vi "Treat Command.vi"(8 "error in (no error)":errorcluster, 11 "Channel in":refnum<class "Channel.lvclass">) -> (0 "error out":errorcluster, 3 "Channel out":refnum<class "Channel.lvclass">)   [LabVIEW 2018, in "Channel.lvclass"]
uses:
  Channel.lvclass
  Channel.lvclass/Channel.ctl
  CCDCamera/CCDCamera.lvclass/CCDCamera.ctl
  Cooler/Cooler.lvclass/Cooler.ctl
  Save Image/Save Image.lvclass/Save Image.ctl
  CCDCamera/CCDCamera.lvclass
  Cooler/Cooler.lvclass
  State Machine/State Machine.lvclass
  RxTx/RxTx.lvclass
  Image Constructor/Image Constructor.lvclass
  Interface/Interface.lvclass
  Save Image/Save Image.lvclass
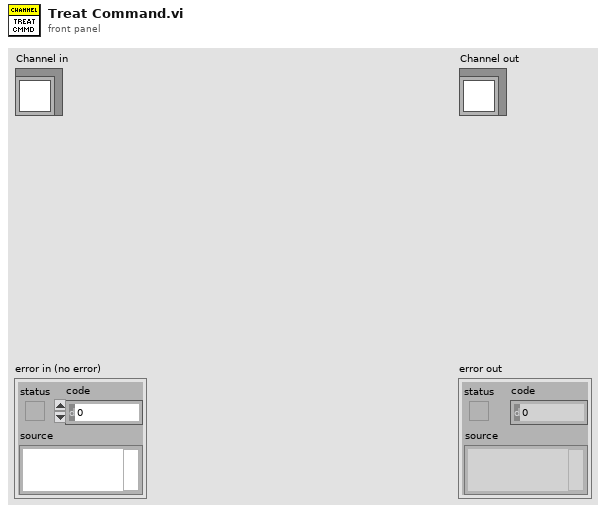
[diagram p1: front panel]
types:
  T1 = cluster{"Initialization":bool, "Serial Number":u16}
  T2 = cluster{"Current Temperature":i16, "Temperatue Status":string}
  T3 = cluster{"Exposure Time":sgl, "Pre-amp gain":u8, "Readout Rate":u8, "EM Mode":u8, "EM Gain":u16, "Binning":u16, "Initial Line":u16, "Initial Cloumn":u16, "Final Line":u16, "Final Column":u16, "Kinetic Series Length":u32, "Shutter Mode":u8, "Cooler ON/OFF":u16, "Temperature":i8, "Image Name":string, "Image Path":string, "# Images":u32}
  T4 = cluster{"Image Path":string, "Image Name":string, "Exposure Time":sgl, "Pre-amp gain":u8, "Readout Rate":u8, "EM Mode":u8, "EM Gain":u16, "Binning":u16, "Initial Line":u16, "Initial Cloumn":u16, "Final Line":u16, "Final Column":u16, "Kinetic Series Length":u32, "Shutter Mode":u8, "Cooler ON/OFF":u16, "Temperature":i8}
  T5 = cluster{"Initial Line":u16, "Initial Column":u16, "Final Line ":u16, "Final Column":u16, "Binning":u16, "Kinetic Series Length":u16, "Image Name":string, "Image Path":string}
  T6 = cluster{"Exposure Time":sgl, "EM Gain":u16, "Binning":u16, "Initial Line":u16, "Initial Cloumn":u16, "Final Line":u16, "Final Column":u16, "Kinetic Series Length":u32, "Shutter Mode":u8, "Pre-amp gain":u8, "Readout Rate":u8, "EM Mode":u8}
  T7 = cluster{"Exposure Time":sgl, "Pre-amp gain":u8, "Readout Rate":u8, "EM Mode":u8, "EM Gain":u16, "Binning":u16, "Initial Line":u16, "Initial Cloumn":u16, "Final Line":u16, "Final Column":u16, "Kinetic Series Length":u32, "Shutter Mode":u8, "Cooler ON/OFF":u16, "Temperature":i8, "Image Name":string, "Image Path":string, "#Images":u32}
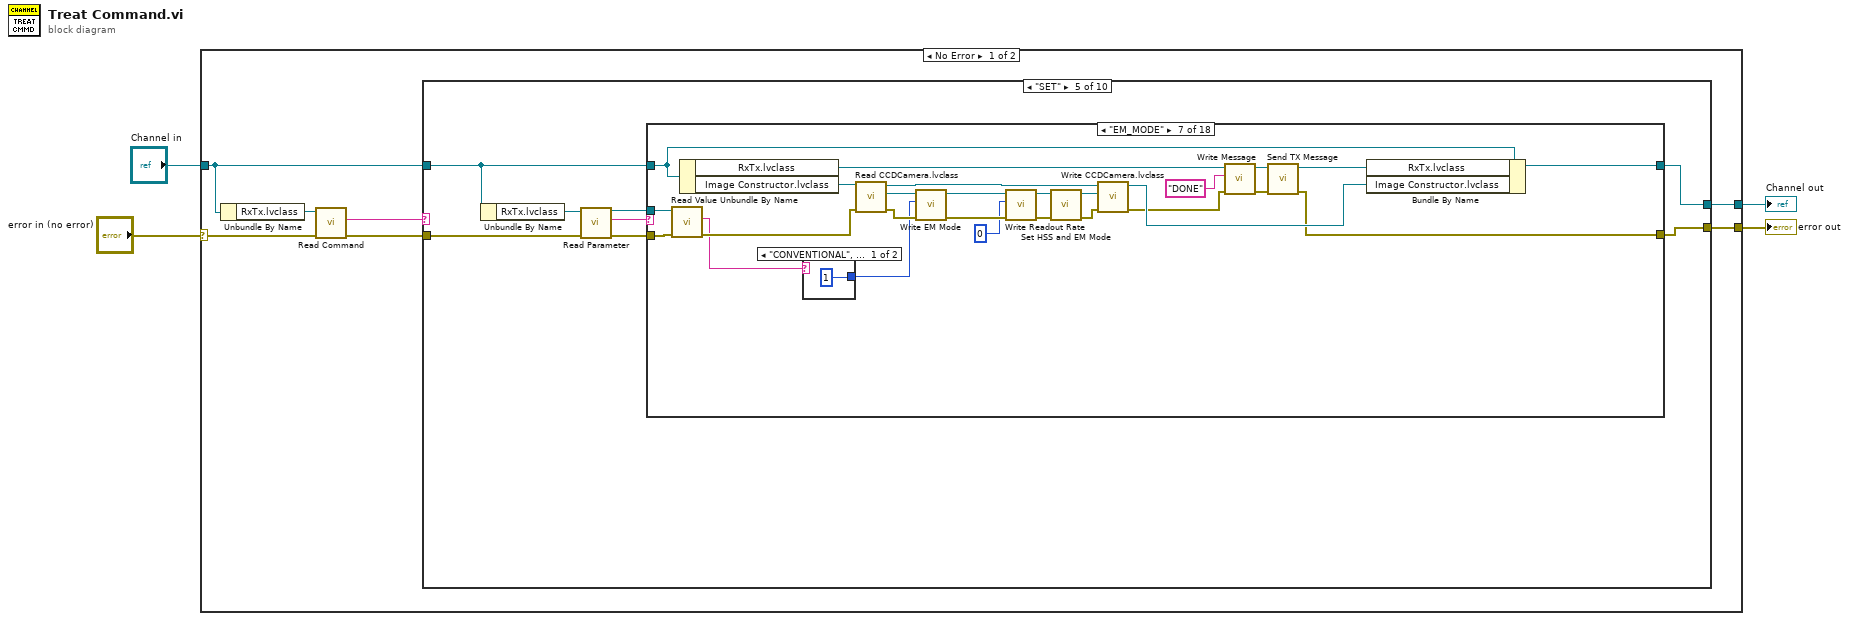
[diagram p0: block diagram]
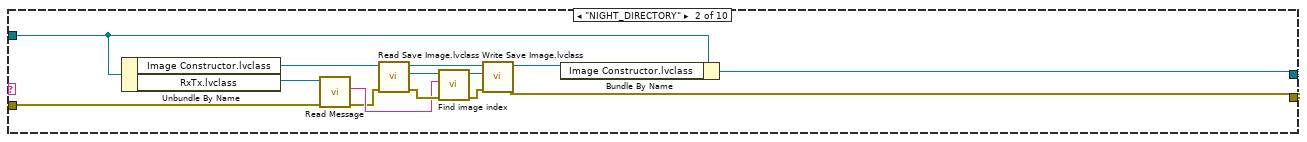
[diagram p3: hidden frame]
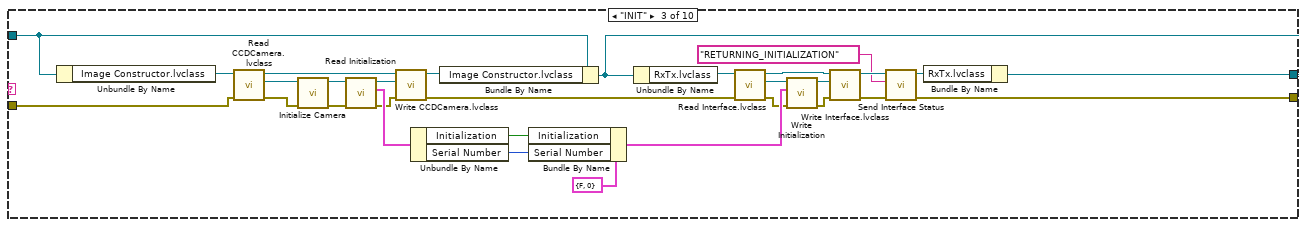
[diagram p4: hidden frame]
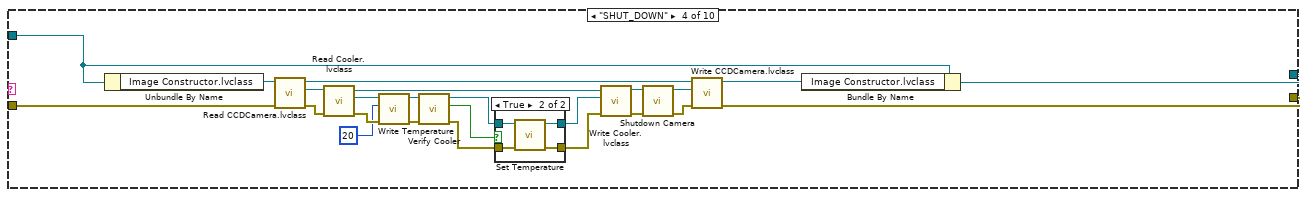
[diagram p5: hidden frame]
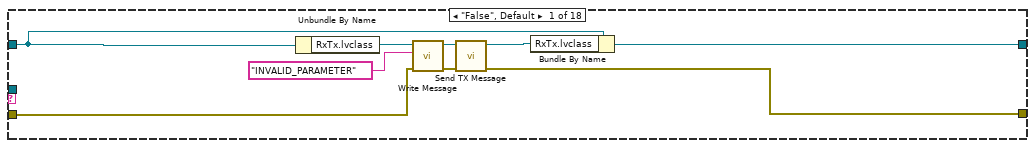
[diagram p7: hidden frame]
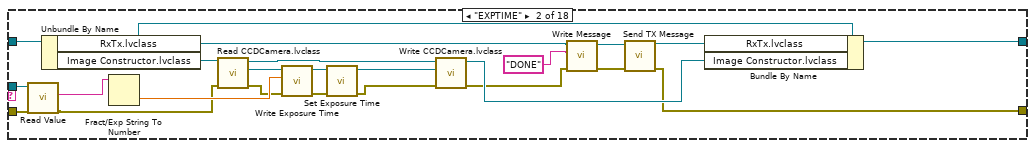
[diagram p8: hidden frame]
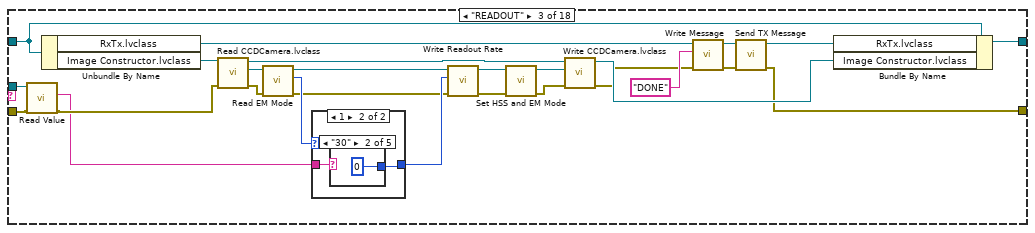
[diagram p9: hidden frame]
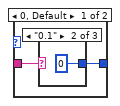
[diagram p10: hidden frame]
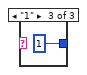
[diagram p12: hidden frame]
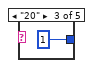
[diagram p14: hidden frame]
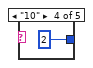
[diagram p15: hidden frame]
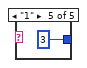
[diagram p16: hidden frame]
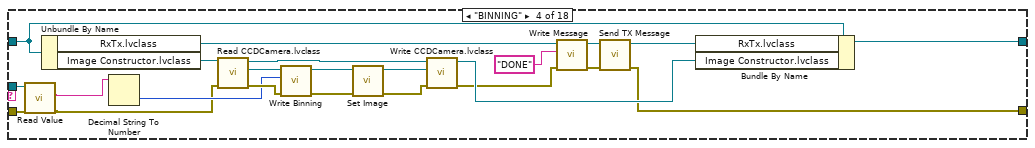
[diagram p17: hidden frame]
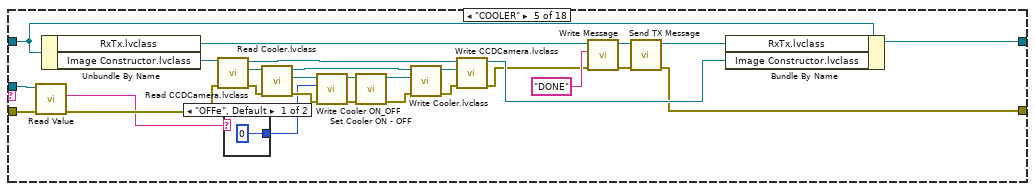
[diagram p18: hidden frame]
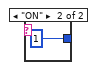
[diagram p19: hidden frame]
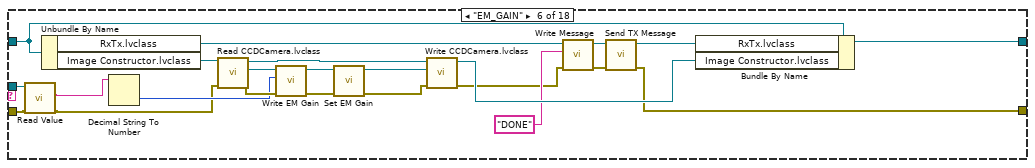
[diagram p20: hidden frame]
diagram:
  n1 = case shown="No Error" "error in (no error)" {
    selector: "error in (no error)" -> [w10 w888]
    tunnel: [w5 w888] -> w3
    tunnel: [w7 w887] -> w1
    tunnel: "Channel in" -> [w8 w887]
    frame No Error {
      n2 = Unbundle By Name(w8) -> ("RxTx.lvclass"=w11:refnum<class "RxTx.lvclass">)
      n3 = call "Read Command.vi"("error in (no error)"=w10, "RxTx in"=w11) -> ("error out"=w6:errorcluster, "Command"=w9:string)  [unwired: 7 in, 1 out]
      n4 = case shown="\"SET\"" w9 {
        tunnel: w8 -> [w13 w16 w31 w60 w90 w518 w769 w802 w841 w885]
        tunnel: [w13 w14 w29 w59 w89 w516 w766 w801 w839 w883] -> w7
        tunnel: w6 -> [w12 w17 w30 w61 w91 w517 w767 w803 w840 w881]
        tunnel: [w12 w15 w28 w58 w88 w515 w765 w800 w838 w882] -> w5
        frame "False", Default {
        }
        frame "NIGHT_DIRECTORY" {
          n5 = Unbundle By Name(w16) -> ("Image Constructor.lvclass"=w26:refnum<class "Image Constructor.lvclass">, "RxTx.lvclass"=w22:refnum<class "RxTx.lvclass">)
          n6 = call "Read Message.vi"("error in (no error)"=w17, "RxTx in"=w22) -> ("error out"=w20:errorcluster, "Message"=w21:string)  [unwired: 7 in, 1 out]
          n7 = call "Read Save Image.lvclass.vi"("error in (no error)"=w20, "Image Constructor in"=w26) -> ("error out"=w24:errorcluster, "Save Image.lvclass"=w23:refnum<class "Save Image.lvclass">, "Image Constructor out"=w27:refnum<class "Image Constructor.lvclass">)  [unwired: 7 in]
          n8 = call "Find image index.vi"("error in (no error)"=w24, "Message"=w21, "Save Image in"=w23) -> ("error out"=w25:errorcluster, "Save Image in"=w19:refnum<class "Save Image.lvclass">)  [unwired: 7 in]
          n9 = call "Write Save Image.lvclass.vi"("error in (no error)"=w25, "Save Image.lvclass"=w19, "Image Constructor in"=w27) -> ("error out"=w15:errorcluster, "Image Constructor out"=w18:refnum<class "Image Constructor.lvclass">)  [unwired: 7 in]
          n10 = Bundle By Name(cluster=w16, "Image Constructor.lvclass"=w18) -> (w14:refnum<class "Channel.lvclass">)
        }
        frame "INIT" {
          n11 = Unbundle By Name(w31) -> ("Image Constructor.lvclass"=w45:refnum<class "Image Constructor.lvclass">)
          n12 = call "Read CCDCamera.lvclass.vi"("error in (no error)"=w30, "Image Constructor in"=w45) -> ("error out"=w47:errorcluster, "CCDCamera.lvclass"=w46:refnum<class "CCDCamera.lvclass">, "Image Constructor out"=w57:refnum<class "Image Constructor.lvclass">)  [unwired: 7 in]
          n13 = call "Initialize Camera.vi"("error in (no error)"=w47, "CCDCamera in"=w46) -> ("error out"=w43:errorcluster, "CCDCamera out"=w44:refnum<class "CCDCamera.lvclass">)  [unwired: 8 in]
          n14 = call "Read Initialization.vi"("error in (no error)"=w43, "CCDCamera in"=w44) -> ("error out"=w52:errorcluster, "Initialization"=w54:T1, "CCDCamera out"=w53:refnum<class "CCDCamera.lvclass">)  [unwired: 7 in]
          n15 = call "Write CCDCamera.lvclass.vi"("error in (no error)"=w52, "CCDCamera.lvclass"=w53, "Image Constructor in"=w57) -> ("error out"=w42:errorcluster, "Image Constructor out"=w56:refnum<class "Image Constructor.lvclass">)  [unwired: 7 in]
          n16 = Unbundle By Name(w54) -> ("Initialization"=w49:bool, "Serial Number"=w48:u16)
          n17 = Bundle By Name(cluster=w31, "Image Constructor.lvclass"=w56) -> (w55:refnum<class "Channel.lvclass">)
          n18 = Bundle By Name(cluster=T1 {"Initialization"=FALSE, "Serial Number"=0} ("Initialization"), "Initialization"=w49, "Serial Number"=w48) -> (w51:T1)
          n19 = Unbundle By Name(w55) -> ("RxTx.lvclass"=w38:refnum<class "RxTx.lvclass">)
          n20 = call "Read Interface.lvclass.vi"("error in (no error)"=w42, "RxTx in"=w38) -> ("error out"=w36:errorcluster, "Interface.lvclass"=w40:refnum<class "Interface.lvclass">, "RxTx out"=w37:refnum<class "RxTx.lvclass">)  [unwired: 7 in]
          n21 = call "Write Initialization.vi"("error in (no error)"=w36, "Initialization"=w51, "Interface in"=w40) -> ("error out"=w41:errorcluster, "Interface out"=w39:refnum<class "Interface.lvclass">)  [unwired: 7 in]
          n22 = call "Write Interface.lvclass.vi"("error in (no error)"=w41, "Interface.lvclass"=w39, "RxTx in"=w37) -> ("error out"=w33:errorcluster, "RxTx out"=w34:refnum<class "RxTx.lvclass">)  [unwired: 7 in]
          n23 = call "Send Interface Status.vi"("error in (no error)"=w33, "Message"="RETURNING_INITIALIZATION", "RxTx in"=w34) -> ("error out"=w28:errorcluster, "RxTx out"=w35:refnum<class "RxTx.lvclass">)  [unwired: 7 in]
          n24 = Bundle By Name(cluster=w55, "RxTx.lvclass"=w35) -> (w29:refnum<class "Channel.lvclass">)
        }
        frame "SHUT_DOWN" {
          n25 = Unbundle By Name(w60) -> ("Image Constructor.lvclass"=w63:refnum<class "Image Constructor.lvclass">)
          n26 = call "Read CCDCamera.lvclass.vi"("error in (no error)"=w61, "Image Constructor in"=w63) -> ("error out"=w65:errorcluster, "CCDCamera.lvclass"=w64:refnum<class "CCDCamera.lvclass">, "Image Constructor out"=w80:refnum<class "Image Constructor.lvclass">)  [unwired: 7 in]
          n27 = call-dynamic "Read Cooler.lvclass.vi"("error in (no error)"=w65, "CCDCamera in"=w64) -> ("error out"=w68:errorcluster, "Cooler.lvclass"=w67:refnum<class "Cooler.lvclass">, "CCDCamera out"=w66:refnum<class "CCDCamera.lvclass">)  [unwired: 7 in]
          n28 = call-dynamic "Write Temperature.vi"("error in (no error)"=w68, "Temperature"=20, "Cooler in"=w67) -> ("error out"=w70:errorcluster, "Cooler out"=w69:refnum<class "Cooler.lvclass">)  [unwired: 7 in]
          n29 = call "Verify Cooler.vi"("error in (no error)"=w70, "Cooler in"=w69) -> ("error out"=w73:errorcluster, "coolerStatus"=w71:bool, "Cooler out"=w72:refnum<class "Cooler.lvclass">)  [unwired: 7 in]
          n30 = case shown="True" w71 {
            tunnel: w72 -> [w83 w87]
            tunnel: w73 -> [w82 w86]
            tunnel: [w82 w85] -> w75
            tunnel: [w83 w84] -> w74
            frame False {
            }
            frame True {
              n31 = call "Set Temperature.vi"("error in (no error)"=w86, "Cooler in"=w87) -> ("error out"=w85:errorcluster, "Cooler out"=w84:refnum<class "Cooler.lvclass">)  [unwired: 8 in]
            }
          }
          n32 = call-dynamic "Write Cooler.lvclass.vi"("error in (no error)"=w75, "Cooler.lvclass"=w74, "CCDCamera in"=w66) -> ("error out"=w76:errorcluster, "CCDCamera out"=w77:refnum<class "CCDCamera.lvclass">)  [unwired: 7 in]
          n33 = call "Shutdown Camera.vi"("error in (no error)"=w76, "CCDCamera in"=w77) -> ("error out"=w79:errorcluster, "CCDCamera out"=w78:refnum<class "CCDCamera.lvclass">)  [unwired: 8 in]
          n34 = call "Write CCDCamera.lvclass.vi"("error in (no error)"=w79, "CCDCamera.lvclass"=w78, "Image Constructor in"=w80) -> ("error out"=w58:errorcluster, "Image Constructor out"=w81:refnum<class "Image Constructor.lvclass">)  [unwired: 7 in]
          n35 = Bundle By Name(cluster=w60, "Image Constructor.lvclass"=w81) -> (w59:refnum<class "Channel.lvclass">)
        }
        frame "SET" {
          n36 = Unbundle By Name(w90) -> ("RxTx.lvclass"=w92:refnum<class "RxTx.lvclass">)
          n37 = call "Read Parameter.vi"("error in (no error)"=w91, "RxTx in"=w92) -> ("error out"=w94:errorcluster, "Parameter"=w93:string, "RxTx out"=w95:refnum<class "RxTx.lvclass">)  [unwired: 7 in]
          n38 = case shown="\"EM_MODE\"" w93 {
            tunnel: [w103 w127 w153 w186 w214 w239 w265 w290 w313 w336 w359 w379 w399 w427 w451 w477 w500 w504] -> w89
            tunnel: w90 -> [w104 w126 w152 w185 w213 w238 w264 w289 w312 w335 w358 w378 w398 w426 w450 w476 w499 w512]
            tunnel: [w98 w109 w142 w169 w202 w225 w252 w274 w297 w322 w344 w367 w389 w417 w438 w463 w486 w501] -> w88
            tunnel: w94 -> [w97 w119 w148 w178 w209 w231 w258 w282 w305 w328 w351 w374 w393 w422 w444 w468 w492 w513]
            tunnel: w95 -> [_ w117 w147 w177 w207 w230 w257 w281 w304 w327 w350 w373 w394 w421 w443 w469 w491 w514]
            frame "False", Default {
              n39 = Unbundle By Name(w104) -> ("RxTx.lvclass"=w100:refnum<class "RxTx.lvclass">)
              n40 = call "Write Message.vi"("error in (no error)"=w97, "Message"="INVALID_PARAMETER", "RxTx in"=w100) -> ("error out"=w102:errorcluster, "RxTx out"=w101:refnum<class "RxTx.lvclass">)  [unwired: 7 in]
              n41 = call "Send TX Message.vi"("error in (no error)"=w102, "RxTx in"=w101) -> ("error out"=w98:errorcluster, "RxTx out"=w99:refnum<class "RxTx.lvclass">)  [unwired: 8 in]
              n42 = Bundle By Name(cluster=w104, "RxTx.lvclass"=w99) -> (w103:refnum<class "Channel.lvclass">)
            }
            frame "EXPTIME" {
              n43 = call "Read Value.vi"("error in (no error)"=w119, "RxTx in"=w117) -> ("error out"=w118:errorcluster, "Value"=w116:string)  [unwired: 7 in, 1 out]
              n44 = Unbundle By Name(w126) -> ("RxTx.lvclass"=w115:refnum<class "RxTx.lvclass">, "Image Constructor.lvclass"=w125:refnum<class "Image Constructor.lvclass">)
              n45 = Fract/Exp String To Number(string=w116) -> (number=w123:dbl)  [unwired: 3 in, 1 out]
              n46 = call "Read CCDCamera.lvclass.vi"("error in (no error)"=w118, "Image Constructor in"=w125) -> ("error out"=w122:errorcluster, "CCDCamera.lvclass"=w124:refnum<class "CCDCamera.lvclass">, "Image Constructor out"=w121:refnum<class "Image Constructor.lvclass">)  [unwired: 7 in]
              n47 = call "Write Exposure Time.vi"("error in (no error)"=w122, "Exposure Time"=w123, "CCDCamera in"=w124) -> ("error out"=w106:errorcluster, "CCDCamera out"=w108:refnum<class "CCDCamera.lvclass">)  [unwired: 7 in]
              n48 = call "Set Exposure Time.vi"("error in (no error)"=w106, "CCDCamera in"=w108) -> ("error out"=w105:errorcluster, "CCDCamera out"=w107:refnum<class "CCDCamera.lvclass">)  [unwired: 8 in]
              n49 = call "Write CCDCamera.lvclass.vi"("error in (no error)"=w105, "CCDCamera.lvclass"=w107, "Image Constructor in"=w121) -> ("error out"=w114:errorcluster, "Image Constructor out"=w120:refnum<class "Image Constructor.lvclass">)  [unwired: 7 in]
              n50 = call "Write Message.vi"("error in (no error)"=w114, "Message"="DONE", "RxTx in"=w115) -> ("error out"=w112:errorcluster, "RxTx out"=w111:refnum<class "RxTx.lvclass">)  [unwired: 7 in]
              n51 = call "Send TX Message.vi"("error in (no error)"=w112, "RxTx in"=w111) -> ("error out"=w109:errorcluster, "RxTx out"=w110:refnum<class "RxTx.lvclass">)  [unwired: 8 in]
              n52 = Bundle By Name(cluster=w126, "RxTx.lvclass"=w110, "Image Constructor.lvclass"=w120) -> (w127:refnum<class "Channel.lvclass">)
            }
            frame "READOUT" {
              n53 = call "Read Value.vi"("error in (no error)"=w148, "RxTx in"=w147) -> ("error out"=w146:errorcluster, "Value"=w131:string)  [unwired: 7 in, 1 out]
              n54 = Unbundle By Name(w152) -> ("RxTx.lvclass"=w140:refnum<class "RxTx.lvclass">, "Image Constructor.lvclass"=w151:refnum<class "Image Constructor.lvclass">)
              n55 = call "Read CCDCamera.lvclass.vi"("error in (no error)"=w146, "Image Constructor in"=w151) -> ("error out"=w133:errorcluster, "CCDCamera.lvclass"=w134:refnum<class "CCDCamera.lvclass">, "Image Constructor out"=w150:refnum<class "Image Constructor.lvclass">)  [unwired: 7 in]
              n56 = call "Read EM Mode.vi"("error in (no error)"=w133, "CCDCamera in"=w134) -> ("error out"=w129:errorcluster, "EM Mode"=w132:u8, "CCDCamera out"=w128:refnum<class "CCDCamera.lvclass">)  [unwired: 7 in]
              n57 = case shown="1" w132 {
                tunnel: w131 -> [w155 w159]
                tunnel: [w154 w158] -> w130
                frame 0, Default {
                  n58 = case shown="\"0.1\"" w155 {
                    tunnel: [_ 0 1] -> w154
                    frame "False", Default {
                    }
                    frame "0.1" {
                    }
                    frame "1" {
                    }
                  }
                }
                frame 1 {
                  n59 = case shown="\"30\"" w159 {
                    tunnel: [_ 0 1 2 3] -> w158
                    frame "False", Default {
                    }
                    frame "30" {
                    }
                    frame "20" {
                    }
                    frame "10" {
                    }
                    frame "1" {
                    }
                  }
                }
              }
              n60 = call "Write Readout Rate.vi"("error in (no error)"=w129, "Readout Rate"=w130, "CCDCamera in"=w128) -> ("error out"=w137:errorcluster, "CCDCamera out"=w138:refnum<class "CCDCamera.lvclass">)  [unwired: 7 in]
              n61 = call "Set HSS and EM Mode.vi"("error in (no error)"=w137, "CCDCamera in"=w138) -> ("error out"=w136:errorcluster, "CCDCamera out"=w135:refnum<class "CCDCamera.lvclass">)  [unwired: 8 in]
              n62 = call "Write CCDCamera.lvclass.vi"("error in (no error)"=w136, "CCDCamera.lvclass"=w135, "Image Constructor in"=w150) -> ("error out"=w139:errorcluster, "Image Constructor out"=w149:refnum<class "Image Constructor.lvclass">)  [unwired: 7 in]
              n63 = call "Write Message.vi"("error in (no error)"=w139, "Message"="DONE", "RxTx in"=w140) -> ("error out"=w141:errorcluster, "RxTx out"=w145:refnum<class "RxTx.lvclass">)  [unwired: 7 in]
              n64 = call "Send TX Message.vi"("error in (no error)"=w141, "RxTx in"=w145) -> ("error out"=w142:errorcluster, "RxTx out"=w143:refnum<class "RxTx.lvclass">)  [unwired: 8 in]
              n65 = Bundle By Name(cluster=w152, "RxTx.lvclass"=w143, "Image Constructor.lvclass"=w149) -> (w153:refnum<class "Channel.lvclass">)
            }
            frame "BINNING" {
              n66 = call "Read Value.vi"("error in (no error)"=w178, "RxTx in"=w177) -> ("error out"=w176:errorcluster, "Value"=w175:string)  [unwired: 7 in, 1 out]
              n67 = Unbundle By Name(w185) -> ("RxTx.lvclass"=w171:refnum<class "RxTx.lvclass">, "Image Constructor.lvclass"=w184:refnum<class "Image Constructor.lvclass">)
              n68 = Decimal String To Number(string=w175) -> (number=w179:i32)  [unwired: 2 in, 1 out]
              n69 = call "Read CCDCamera.lvclass.vi"("error in (no error)"=w176, "Image Constructor in"=w184) -> ("error out"=w180:errorcluster, "CCDCamera.lvclass"=w181:refnum<class "CCDCamera.lvclass">, "Image Constructor out"=w183:refnum<class "Image Constructor.lvclass">)  [unwired: 7 in]
              n70 = call "Write Binning.vi"("error in (no error)"=w180, "Binning"=w179, "CCDCamera in"=w181) -> ("error out"=w164:errorcluster, "CCDCamera out"=w167:refnum<class "CCDCamera.lvclass">)  [unwired: 7 in]
              n71 = call "Set Image.vi"("error in (no error)"=w164, "CCDCamera in"=w167) -> ("error out"=w165:errorcluster, "CCDCamera out"=w166:refnum<class "CCDCamera.lvclass">)  [unwired: 8 in]
              n72 = call "Write CCDCamera.lvclass.vi"("error in (no error)"=w165, "CCDCamera.lvclass"=w166, "Image Constructor in"=w183) -> ("error out"=w168:errorcluster, "Image Constructor out"=w182:refnum<class "Image Constructor.lvclass">)  [unwired: 7 in]
              n73 = call "Write Message.vi"("error in (no error)"=w168, "Message"="DONE", "RxTx in"=w171) -> ("error out"=w174:errorcluster, "RxTx out"=w173:refnum<class "RxTx.lvclass">)  [unwired: 7 in]
              n74 = call "Send TX Message.vi"("error in (no error)"=w174, "RxTx in"=w173) -> ("error out"=w169:errorcluster, "RxTx out"=w170:refnum<class "RxTx.lvclass">)  [unwired: 8 in]
              n75 = Bundle By Name(cluster=w185, "RxTx.lvclass"=w170, "Image Constructor.lvclass"=w182) -> (w186:refnum<class "Channel.lvclass">)
            }
            frame "COOLER" {
              n76 = call "Read Value.vi"("error in (no error)"=w209, "RxTx in"=w207) -> ("error out"=w208:errorcluster, "Value"=w188:string)  [unwired: 7 in, 1 out]
              n77 = Unbundle By Name(w213) -> ("RxTx.lvclass"=w204:refnum<class "RxTx.lvclass">, "Image Constructor.lvclass"=w212:refnum<class "Image Constructor.lvclass">)
              n78 = call "Read CCDCamera.lvclass.vi"("error in (no error)"=w208, "Image Constructor in"=w212) -> ("error out"=w198:errorcluster, "CCDCamera.lvclass"=w199:refnum<class "CCDCamera.lvclass">, "Image Constructor out"=w211:refnum<class "Image Constructor.lvclass">)  [unwired: 7 in]
              n79 = case shown="\"OFFe\", Default" w188 {
                tunnel: [0 1] -> w187
                frame "OFFe", Default {
                }
                frame "ON" {
                }
              }
              n80 = call-dynamic "Read Cooler.lvclass.vi"("error in (no error)"=w198, "CCDCamera in"=w199) -> ("error out"=w190:errorcluster, "Cooler.lvclass"=w191:refnum<class "Cooler.lvclass">, "CCDCamera out"=w189:refnum<class "CCDCamera.lvclass">)  [unwired: 7 in]
              n81 = call "Write Cooler ON_OFF.vi"("error in (no error)"=w190, "Cooler ON/OFF"=w187, "Cooler in"=w191) -> ("error out"=w192:errorcluster, "Cooler out"=w193:refnum<class "Cooler.lvclass">)  [unwired: 7 in]
              n82 = call "Set Cooler ON - OFF.vi"("error in (no error)"=w192, "Cooler in"=w193) -> ("error out"=w194:errorcluster, "Cooler out"=w195:refnum<class "Cooler.lvclass">)  [unwired: 8 in]
              n83 = call-dynamic "Write Cooler.lvclass.vi"("error in (no error)"=w194, "Cooler.lvclass"=w195, "CCDCamera in"=w189) -> ("error out"=w196:errorcluster, "CCDCamera out"=w197:refnum<class "CCDCamera.lvclass">)  [unwired: 7 in]
              n84 = call "Write CCDCamera.lvclass.vi"("error in (no error)"=w196, "CCDCamera.lvclass"=w197, "Image Constructor in"=w211) -> ("error out"=w200:errorcluster, "Image Constructor out"=w210:refnum<class "Image Constructor.lvclass">)  [unwired: 7 in]
              n85 = call "Write Message.vi"("error in (no error)"=w200, "Message"="DONE", "RxTx in"=w204) -> ("error out"=w206:errorcluster, "RxTx out"=w205:refnum<class "RxTx.lvclass">)  [unwired: 7 in]
              n86 = call "Send TX Message.vi"("error in (no error)"=w206, "RxTx in"=w205) -> ("error out"=w202:errorcluster, "RxTx out"=w203:refnum<class "RxTx.lvclass">)  [unwired: 8 in]
              n87 = Bundle By Name(cluster=w213, "RxTx.lvclass"=w203, "Image Constructor.lvclass"=w210) -> (w214:refnum<class "Channel.lvclass">)
            }
            frame "EM_GAIN" {
              n88 = call "Read Value.vi"("error in (no error)"=w231, "RxTx in"=w230) -> ("error out"=w229:errorcluster, "Value"=w228:string)  [unwired: 7 in, 1 out]
              n89 = Unbundle By Name(w238) -> ("RxTx.lvclass"=w223:refnum<class "RxTx.lvclass">, "Image Constructor.lvclass"=w237:refnum<class "Image Constructor.lvclass">)
              n90 = Decimal String To Number(string=w228) -> (number=w232:i32)  [unwired: 2 in, 1 out]
              n91 = call "Read CCDCamera.lvclass.vi"("error in (no error)"=w229, "Image Constructor in"=w237) -> ("error out"=w233:errorcluster, "CCDCamera.lvclass"=w234:refnum<class "CCDCamera.lvclass">, "Image Constructor out"=w236:refnum<class "Image Constructor.lvclass">)  [unwired: 7 in]
              n92 = call "Write EM Gain.vi"("error in (no error)"=w233, "EM Gain"=w232, "CCDCamera in"=w234) -> ("error out"=w220:errorcluster, "CCDCamera out"=w219:refnum<class "CCDCamera.lvclass">)  [unwired: 7 in]
              n93 = call "Set EM Gain.vi"("error in (no error)"=w220, "CCDCamera in"=w219) -> ("error out"=w217:errorcluster, "CCDCamera out"=w218:refnum<class "CCDCamera.lvclass">)  [unwired: 8 in]
              n94 = call "Write CCDCamera.lvclass.vi"("error in (no error)"=w217, "CCDCamera.lvclass"=w218, "Image Constructor in"=w236) -> ("error out"=w221:errorcluster, "Image Constructor out"=w235:refnum<class "Image Constructor.lvclass">)  [unwired: 7 in]
              n95 = call "Write Message.vi"("error in (no error)"=w221, "Message"="DONE", "RxTx in"=w223) -> ("error out"=w227:errorcluster, "RxTx out"=w226:refnum<class "RxTx.lvclass">)  [unwired: 7 in]
              n96 = call "Send TX Message.vi"("error in (no error)"=w227, "RxTx in"=w226) -> ("error out"=w225:errorcluster, "RxTx out"=w224:refnum<class "RxTx.lvclass">)  [unwired: 8 in]
              n97 = Bundle By Name(cluster=w238, "RxTx.lvclass"=w224, "Image Constructor.lvclass"=w235) -> (w239:refnum<class "Channel.lvclass">)
            }
            frame "EM_MODE" {
              n98 = call "Read Value.vi"("error in (no error)"=w258, "RxTx in"=w257) -> ("error out"=w256:errorcluster, "Value"=w246:string)  [unwired: 7 in, 1 out]
              n99 = Unbundle By Name(w264) -> ("RxTx.lvclass"=w250:refnum<class "RxTx.lvclass">, "Image Constructor.lvclass"=w263:refnum<class "Image Constructor.lvclass">)
              n100 = case shown="\"CONVENTIONAL\", Default" w246 {
                tunnel: [1 0] -> w245
                frame "CONVENTIONAL", Default {
                }
                frame "EM" {
                }
              }
              n101 = call "Read CCDCamera.lvclass.vi"("error in (no error)"=w256, "Image Constructor in"=w263) -> ("error out"=w259:errorcluster, "CCDCamera.lvclass"=w260:refnum<class "CCDCamera.lvclass">, "Image Constructor out"=w262:refnum<class "Image Constructor.lvclass">)  [unwired: 7 in]
              n102 = call "Write EM Mode.vi"("error in (no error)"=w259, "EM Mode"=w245, "CCDCamera in"=w260) -> ("error out"=w241:errorcluster, "CCDCamera out"=w244:refnum<class "CCDCamera.lvclass">)  [unwired: 7 in]
              n103 = call "Write Readout Rate.vi"("error in (no error)"=w241, "Readout Rate"=0, "CCDCamera in"=w244) -> ("error out"=w242:errorcluster, "CCDCamera out"=w243:refnum<class "CCDCamera.lvclass">)  [unwired: 7 in]
              n104 = call "Set HSS and EM Mode.vi"("error in (no error)"=w242, "CCDCamera in"=w243) -> ("error out"=w247:errorcluster, "CCDCamera out"=w248:refnum<class "CCDCamera.lvclass">)  [unwired: 8 in]
              n105 = call "Write CCDCamera.lvclass.vi"("error in (no error)"=w247, "CCDCamera.lvclass"=w248, "Image Constructor in"=w262) -> ("error out"=w251:errorcluster, "Image Constructor out"=w261:refnum<class "Image Constructor.lvclass">)  [unwired: 7 in]
              n106 = call "Write Message.vi"("error in (no error)"=w251, "Message"="DONE", "RxTx in"=w250) -> ("error out"=w255:errorcluster, "RxTx out"=w254:refnum<class "RxTx.lvclass">)  [unwired: 7 in]
              n107 = call "Send TX Message.vi"("error in (no error)"=w255, "RxTx in"=w254) -> ("error out"=w252:errorcluster, "RxTx out"=w253:refnum<class "RxTx.lvclass">)  [unwired: 8 in]
              n108 = Bundle By Name(cluster=w264, "RxTx.lvclass"=w253, "Image Constructor.lvclass"=w261) -> (w265:refnum<class "Channel.lvclass">)
            }
            frame "FINAL_COLUMN" {
              n109 = call "Read Value.vi"("error in (no error)"=w282, "RxTx in"=w281) -> ("error out"=w280:errorcluster, "Value"=w279:string)  [unwired: 7 in, 1 out]
              n110 = Unbundle By Name(w289) -> ("RxTx.lvclass"=w276:refnum<class "RxTx.lvclass">, "Image Constructor.lvclass"=w288:refnum<class "Image Constructor.lvclass">)
              n111 = Decimal String To Number(string=w279) -> (number=w283:i32)  [unwired: 2 in, 1 out]
              n112 = call "Read CCDCamera.lvclass.vi"("error in (no error)"=w280, "Image Constructor in"=w288) -> ("error out"=w284:errorcluster, "CCDCamera.lvclass"=w285:refnum<class "CCDCamera.lvclass">, "Image Constructor out"=w287:refnum<class "Image Constructor.lvclass">)  [unwired: 7 in]
              n113 = call "Write Final Column.vi"("error in (no error)"=w284, "Final Column"=w283, "CCDCamera in"=w285) -> ("error out"=w270:errorcluster, "CCDCamera out"=w271:refnum<class "CCDCamera.lvclass">)  [unwired: 7 in]
              n114 = call "Set Image.vi"("error in (no error)"=w270, "CCDCamera in"=w271) -> ("error out"=w268:errorcluster, "CCDCamera out"=w269:refnum<class "CCDCamera.lvclass">)  [unwired: 8 in]
              n115 = call "Write CCDCamera.lvclass.vi"("error in (no error)"=w268, "CCDCamera.lvclass"=w269, "Image Constructor in"=w287) -> ("error out"=w273:errorcluster, "Image Constructor out"=w286:refnum<class "Image Constructor.lvclass">)  [unwired: 7 in]
              n116 = call "Write Message.vi"("error in (no error)"=w273, "Message"="DONE", "RxTx in"=w276) -> ("error out"=w278:errorcluster, "RxTx out"=w277:refnum<class "RxTx.lvclass">)  [unwired: 7 in]
              n117 = call "Send TX Message.vi"("error in (no error)"=w278, "RxTx in"=w277) -> ("error out"=w274:errorcluster, "RxTx out"=w275:refnum<class "RxTx.lvclass">)  [unwired: 8 in]
              n118 = Bundle By Name(cluster=w289, "RxTx.lvclass"=w275, "Image Constructor.lvclass"=w286) -> (w290:refnum<class "Channel.lvclass">)
            }
            frame "FINAL_LINE" {
              n119 = call "Read Value.vi"("error in (no error)"=w305, "RxTx in"=w304) -> ("error out"=w303:errorcluster, "Value"=w302:string)  [unwired: 7 in, 1 out]
              n120 = Unbundle By Name(w312) -> ("RxTx.lvclass"=w299:refnum<class "RxTx.lvclass">, "Image Constructor.lvclass"=w311:refnum<class "Image Constructor.lvclass">)
              n121 = Decimal String To Number(string=w302) -> (number=w306:i32)  [unwired: 2 in, 1 out]
              n122 = call "Read CCDCamera.lvclass.vi"("error in (no error)"=w303, "Image Constructor in"=w311) -> ("error out"=w307:errorcluster, "CCDCamera.lvclass"=w308:refnum<class "CCDCamera.lvclass">, "Image Constructor out"=w310:refnum<class "Image Constructor.lvclass">)  [unwired: 7 in]
              n123 = call "Write Final Line.vi"("error in (no error)"=w307, "Final Line"=w306, "CCDCamera in"=w308) -> ("error out"=w293:errorcluster, "CCDCamera out"=w294:refnum<class "CCDCamera.lvclass">)  [unwired: 7 in]
              n124 = call "Set Image.vi"("error in (no error)"=w293, "CCDCamera in"=w294) -> ("error out"=w291:errorcluster, "CCDCamera out"=w292:refnum<class "CCDCamera.lvclass">)  [unwired: 8 in]
              n125 = call "Write CCDCamera.lvclass.vi"("error in (no error)"=w291, "CCDCamera.lvclass"=w292, "Image Constructor in"=w310) -> ("error out"=w296:errorcluster, "Image Constructor out"=w309:refnum<class "Image Constructor.lvclass">)  [unwired: 7 in]
              n126 = call "Write Message.vi"("error in (no error)"=w296, "Message"="DONE", "RxTx in"=w299) -> ("error out"=w301:errorcluster, "RxTx out"=w300:refnum<class "RxTx.lvclass">)  [unwired: 7 in]
              n127 = call "Send TX Message.vi"("error in (no error)"=w301, "RxTx in"=w300) -> ("error out"=w297:errorcluster, "RxTx out"=w298:refnum<class "RxTx.lvclass">)  [unwired: 8 in]
              n128 = Bundle By Name(cluster=w312, "RxTx.lvclass"=w298, "Image Constructor.lvclass"=w309) -> (w313:refnum<class "Channel.lvclass">)
            }
            frame "INITIAL_COLUMN" {
              n129 = call "Read Value.vi"("error in (no error)"=w328, "RxTx in"=w327) -> ("error out"=w326:errorcluster, "Value"=w325:string)  [unwired: 7 in, 1 out]
              n130 = Unbundle By Name(w335) -> ("RxTx.lvclass"=w320:refnum<class "RxTx.lvclass">, "Image Constructor.lvclass"=w334:refnum<class "Image Constructor.lvclass">)
              n131 = Decimal String To Number(string=w325) -> (number=w329:i32)  [unwired: 2 in, 1 out]
              n132 = call "Read CCDCamera.lvclass.vi"("error in (no error)"=w326, "Image Constructor in"=w334) -> ("error out"=w330:errorcluster, "CCDCamera.lvclass"=w331:refnum<class "CCDCamera.lvclass">, "Image Constructor out"=w333:refnum<class "Image Constructor.lvclass">)  [unwired: 7 in]
              n133 = call "Write Initial Cloumn.vi"("error in (no error)"=w330, "Initial Cloumn"=w329, "CCDCamera in"=w331) -> ("error out"=w316:errorcluster, "CCDCamera out"=w317:refnum<class "CCDCamera.lvclass">)  [unwired: 7 in]
              n134 = call "Set Image.vi"("error in (no error)"=w316, "CCDCamera in"=w317) -> ("error out"=w314:errorcluster, "CCDCamera out"=w315:refnum<class "CCDCamera.lvclass">)  [unwired: 8 in]
              n135 = call "Write CCDCamera.lvclass.vi"("error in (no error)"=w314, "CCDCamera.lvclass"=w315, "Image Constructor in"=w333) -> ("error out"=w318:errorcluster, "Image Constructor out"=w332:refnum<class "Image Constructor.lvclass">)  [unwired: 7 in]
              n136 = call "Write Message.vi"("error in (no error)"=w318, "Message"="DONE", "RxTx in"=w320) -> ("error out"=w324:errorcluster, "RxTx out"=w323:refnum<class "RxTx.lvclass">)  [unwired: 7 in]
              n137 = call "Send TX Message.vi"("error in (no error)"=w324, "RxTx in"=w323) -> ("error out"=w322:errorcluster, "RxTx out"=w321:refnum<class "RxTx.lvclass">)  [unwired: 8 in]
              n138 = Bundle By Name(cluster=w335, "RxTx.lvclass"=w321, "Image Constructor.lvclass"=w332) -> (w336:refnum<class "Channel.lvclass">)
            }
            frame "INITIAL_LINE" {
              n139 = call "Read Value.vi"("error in (no error)"=w351, "RxTx in"=w350) -> ("error out"=w349:errorcluster, "Value"=w348:string)  [unwired: 7 in, 1 out]
              n140 = Unbundle By Name(w358) -> ("RxTx.lvclass"=w345:refnum<class "RxTx.lvclass">, "Image Constructor.lvclass"=w357:refnum<class "Image Constructor.lvclass">)
              n141 = Decimal String To Number(string=w348) -> (number=w352:i32)  [unwired: 2 in, 1 out]
              n142 = call "Read CCDCamera.lvclass.vi"("error in (no error)"=w349, "Image Constructor in"=w357) -> ("error out"=w353:errorcluster, "CCDCamera.lvclass"=w354:refnum<class "CCDCamera.lvclass">, "Image Constructor out"=w356:refnum<class "Image Constructor.lvclass">)  [unwired: 7 in]
              n143 = call "Write Initial Line.vi"("error in (no error)"=w353, "Initial Line"=w352, "CCDCamera in"=w354) -> ("error out"=w339:errorcluster, "CCDCamera out"=w340:refnum<class "CCDCamera.lvclass">)  [unwired: 7 in]
              n144 = call "Set Image.vi"("error in (no error)"=w339, "CCDCamera in"=w340) -> ("error out"=w338:errorcluster, "CCDCamera out"=w337:refnum<class "CCDCamera.lvclass">)  [unwired: 8 in]
              n145 = call "Write CCDCamera.lvclass.vi"("error in (no error)"=w338, "CCDCamera.lvclass"=w337, "Image Constructor in"=w356) -> ("error out"=w342:errorcluster, "Image Constructor out"=w355:refnum<class "Image Constructor.lvclass">)  [unwired: 7 in]
              n146 = call "Write Message.vi"("error in (no error)"=w342, "Message"="DONE", "RxTx in"=w345) -> ("error out"=w343:errorcluster, "RxTx out"=w347:refnum<class "RxTx.lvclass">)  [unwired: 7 in]
              n147 = call "Send TX Message.vi"("error in (no error)"=w343, "RxTx in"=w347) -> ("error out"=w344:errorcluster, "RxTx out"=w346:refnum<class "RxTx.lvclass">)  [unwired: 8 in]
              n148 = Bundle By Name(cluster=w358, "RxTx.lvclass"=w346, "Image Constructor.lvclass"=w355) -> (w359:refnum<class "Channel.lvclass">)
            }
            frame "IMAGE_PATH" {
              n149 = call "Read Value.vi"("error in (no error)"=w374, "RxTx in"=w373) -> ("error out"=w372:errorcluster, "Value"=w360:string)  [unwired: 7 in, 1 out]
              n150 = Unbundle By Name(w378) -> ("RxTx.lvclass"=w368:refnum<class "RxTx.lvclass">, "Image Constructor.lvclass"=w377:refnum<class "Image Constructor.lvclass">)
              n151 = call "Read Save Image.lvclass.vi"("error in (no error)"=w372, "Image Constructor in"=w377) -> ("error out"=w361:errorcluster, "Save Image.lvclass"=w362:refnum<class "Save Image.lvclass">, "Image Constructor out"=w376:refnum<class "Image Constructor.lvclass">)  [unwired: 7 in]
              n152 = call "Write Image Path.vi"("error in (no error)"=w361, "Image Path"=w360, "Save Image in"=w362) -> ("error out"=w363:errorcluster, "Save Image out"=w364:refnum<class "Save Image.lvclass">)  [unwired: 7 in]
              n153 = call "Write Save Image.lvclass.vi"("error in (no error)"=w363, "Save Image.lvclass"=w364, "Image Constructor in"=w376) -> ("error out"=w366:errorcluster, "Image Constructor out"=w375:refnum<class "Image Constructor.lvclass">)  [unwired: 7 in]
              n154 = call "Write Message.vi"("error in (no error)"=w366, "Message"="DONE", "RxTx in"=w368) -> ("error out"=w371:errorcluster, "RxTx out"=w370:refnum<class "RxTx.lvclass">)  [unwired: 7 in]
              n155 = call "Send TX Message.vi"("error in (no error)"=w371, "RxTx in"=w370) -> ("error out"=w367:errorcluster, "RxTx out"=w369:refnum<class "RxTx.lvclass">)  [unwired: 8 in]
              n156 = Bundle By Name(cluster=w378, "RxTx.lvclass"=w369, "Image Constructor.lvclass"=w375) -> (w379:refnum<class "Channel.lvclass">)
            }
            frame "IMAGE_NAME" {
              n157 = call "Read Value.vi"("error in (no error)"=w393, "RxTx in"=w394) -> ("error out"=w392:errorcluster, "Value"=w380:string)  [unwired: 7 in, 1 out]
              n158 = Unbundle By Name(w398) -> ("RxTx.lvclass"=w387:refnum<class "RxTx.lvclass">, "Image Constructor.lvclass"=w397:refnum<class "Image Constructor.lvclass">)
              n159 = call "Read Save Image.lvclass.vi"("error in (no error)"=w392, "Image Constructor in"=w397) -> ("error out"=w383:errorcluster, "Save Image.lvclass"=w384:refnum<class "Save Image.lvclass">, "Image Constructor out"=w396:refnum<class "Image Constructor.lvclass">)  [unwired: 7 in]
              n160 = call "Write Image Name.vi"("error in (no error)"=w383, "Image Name"=w380, "Save Image in"=w384) -> ("error out"=w381:errorcluster, "Save Image out"=w382:refnum<class "Save Image.lvclass">)  [unwired: 7 in]
              n161 = call "Write Save Image.lvclass.vi"("error in (no error)"=w381, "Save Image.lvclass"=w382, "Image Constructor in"=w396) -> ("error out"=w386:errorcluster, "Image Constructor out"=w395:refnum<class "Image Constructor.lvclass">)  [unwired: 7 in]
              n162 = call "Write Message.vi"("error in (no error)"=w386, "Message"="DONE", "RxTx in"=w387) -> ("error out"=w391:errorcluster, "RxTx out"=w390:refnum<class "RxTx.lvclass">)  [unwired: 7 in]
              n163 = call "Send TX Message.vi"("error in (no error)"=w391, "RxTx in"=w390) -> ("error out"=w389:errorcluster, "RxTx out"=w388:refnum<class "RxTx.lvclass">)  [unwired: 8 in]
              n164 = Bundle By Name(cluster=w398, "RxTx.lvclass"=w388, "Image Constructor.lvclass"=w395) -> (w399:refnum<class "Channel.lvclass">)
            }
            frame "TEMPERATURE" {
              n165 = call "Read Value.vi"("error in (no error)"=w422, "RxTx in"=w421) -> ("error out"=w420:errorcluster, "Value"=w419:string)  [unwired: 7 in, 1 out]
              n166 = Unbundle By Name(w426) -> ("RxTx.lvclass"=w412:refnum<class "RxTx.lvclass">, "Image Constructor.lvclass"=w425:refnum<class "Image Constructor.lvclass">)
              n167 = Decimal String To Number(string=w419) -> (number=w401:i32)  [unwired: 2 in, 1 out]
              n168 = call "Read CCDCamera.lvclass.vi"("error in (no error)"=w420, "Image Constructor in"=w425) -> ("error out"=w408:errorcluster, "CCDCamera.lvclass"=w409:refnum<class "CCDCamera.lvclass">, "Image Constructor out"=w424:refnum<class "Image Constructor.lvclass">)  [unwired: 7 in]
              n169 = call-dynamic "Read Cooler.lvclass.vi"("error in (no error)"=w408, "CCDCamera in"=w409) -> ("error out"=w406:errorcluster, "Cooler.lvclass"=w407:refnum<class "Cooler.lvclass">, "CCDCamera out"=w400:refnum<class "CCDCamera.lvclass">)  [unwired: 7 in]
              n170 = call-dynamic "Write Temperature.vi"("error in (no error)"=w406, "Temperature"=w401, "Cooler in"=w407) -> ("error out"=w402:errorcluster, "Cooler out"=w403:refnum<class "Cooler.lvclass">)  [unwired: 7 in]
              n171 = call "Set Temperature.vi"("error in (no error)"=w402, "Cooler in"=w403) -> ("error out"=w404:errorcluster, "Cooler out"=w405:refnum<class "Cooler.lvclass">)  [unwired: 8 in]
              n172 = call-dynamic "Write Cooler.lvclass.vi"("error in (no error)"=w404, "Cooler.lvclass"=w405, "CCDCamera in"=w400) -> ("error out"=w410:errorcluster, "CCDCamera out"=w411:refnum<class "CCDCamera.lvclass">)  [unwired: 7 in]
              n173 = call "Write CCDCamera.lvclass.vi"("error in (no error)"=w410, "CCDCamera.lvclass"=w411, "Image Constructor in"=w424) -> ("error out"=w414:errorcluster, "Image Constructor out"=w423:refnum<class "Image Constructor.lvclass">)  [unwired: 7 in]
              n174 = call "Write Message.vi"("error in (no error)"=w414, "Message"="DONE", "RxTx in"=w412) -> ("error out"=w416:errorcluster, "RxTx out"=w418:refnum<class "RxTx.lvclass">)  [unwired: 7 in]
              n175 = call "Send TX Message.vi"("error in (no error)"=w416, "RxTx in"=w418) -> ("error out"=w417:errorcluster, "RxTx out"=w415:refnum<class "RxTx.lvclass">)  [unwired: 8 in]
              n176 = Bundle By Name(cluster=w426, "RxTx.lvclass"=w415, "Image Constructor.lvclass"=w423) -> (w427:refnum<class "Channel.lvclass">)
            }
            frame "SHUTTER" {
              n177 = call "Read Value.vi"("error in (no error)"=w444, "RxTx in"=w443) -> ("error out"=w442:errorcluster, "Value"=w428:string)  [unwired: 7 in, 1 out]
              n178 = Unbundle By Name(w450) -> ("RxTx.lvclass"=w437:refnum<class "RxTx.lvclass">, "Image Constructor.lvclass"=w449:refnum<class "Image Constructor.lvclass">)
              n179 = To Upper Case(1:w428) -> (0:w429:string)
              n180 = case shown="\"CLOSED\", Default" w429 {
                tunnel: [2 1 0] -> w430
                frame "CLOSED", Default {
                }
                frame "OPEN" {
                }
                frame "AUTO" {
                }
              }
              n181 = call "Read CCDCamera.lvclass.vi"("error in (no error)"=w442, "Image Constructor in"=w449) -> ("error out"=w445:errorcluster, "CCDCamera.lvclass"=w446:refnum<class "CCDCamera.lvclass">, "Image Constructor out"=w448:refnum<class "Image Constructor.lvclass">)  [unwired: 7 in]
              n182 = call "Write Shutter Mode.vi"("error in (no error)"=w445, "Shutter Mode"=w430, "CCDCamera in"=w446) -> ("error out"=w433:errorcluster, "CCDCamera out"=w434:refnum<class "CCDCamera.lvclass">)  [unwired: 7 in]
              n183 = call "Set Shutter Mode.vi"("error in (no error)"=w433, "CCDCamera in"=w434) -> ("error out"=w431:errorcluster, "CCDCamera out"=w432:refnum<class "CCDCamera.lvclass">)  [unwired: 8 in]
              n184 = call "Write CCDCamera.lvclass.vi"("error in (no error)"=w431, "CCDCamera.lvclass"=w432, "Image Constructor in"=w448) -> ("error out"=w436:errorcluster, "Image Constructor out"=w447:refnum<class "Image Constructor.lvclass">)  [unwired: 7 in]
              n185 = call "Write Message.vi"("error in (no error)"=w436, "Message"="DONE", "RxTx in"=w437) -> ("error out"=w441:errorcluster, "RxTx out"=w440:refnum<class "RxTx.lvclass">)  [unwired: 7 in]
              n186 = call "Send TX Message.vi"("error in (no error)"=w441, "RxTx in"=w440) -> ("error out"=w438:errorcluster, "RxTx out"=w439:refnum<class "RxTx.lvclass">)  [unwired: 8 in]
              n187 = Bundle By Name(cluster=w450, "RxTx.lvclass"=w439, "Image Constructor.lvclass"=w447) -> (w451:refnum<class "Channel.lvclass">)
            }
            frame "PREAMP" {
              n188 = call "Read Value.vi"("error in (no error)"=w468, "RxTx in"=w469) -> ("error out"=w467:errorcluster, "Value"=w466:string)  [unwired: 7 in, 1 out]
              n189 = Unbundle By Name(w476) -> ("RxTx.lvclass"=w461:refnum<class "RxTx.lvclass">, "Image Constructor.lvclass"=w475:refnum<class "Image Constructor.lvclass">)
              n190 = Decimal String To Number(string=w466) -> (number=w470:i32)  [unwired: 2 in, 1 out]
              n191 = call "Read CCDCamera.lvclass.vi"("error in (no error)"=w467, "Image Constructor in"=w475) -> ("error out"=w471:errorcluster, "CCDCamera.lvclass"=w472:refnum<class "CCDCamera.lvclass">, "Image Constructor out"=w474:refnum<class "Image Constructor.lvclass">)  [unwired: 7 in]
              n192 = call "Write Pre-amp gain.vi"("error in (no error)"=w471, "Pre-amp gain"=w470, "CCDCamera in"=w472) -> ("error out"=w457:errorcluster, "CCDCamera out"=w458:refnum<class "CCDCamera.lvclass">)  [unwired: 7 in]
              n193 = call "Set Pre Amplification.vi"("error in (no error)"=w457, "CCDCamera in"=w458) -> ("error out"=w455:errorcluster, "CCDCamera out"=w456:refnum<class "CCDCamera.lvclass">)  [unwired: 8 in]
              n194 = call "Write CCDCamera.lvclass.vi"("error in (no error)"=w455, "CCDCamera.lvclass"=w456, "Image Constructor in"=w474) -> ("error out"=w460:errorcluster, "Image Constructor out"=w473:refnum<class "Image Constructor.lvclass">)  [unwired: 7 in]
              n195 = call "Write Message.vi"("error in (no error)"=w460, "Message"="DONE", "RxTx in"=w461) -> ("error out"=w465:errorcluster, "RxTx out"=w464:refnum<class "RxTx.lvclass">)  [unwired: 7 in]
              n196 = call "Send TX Message.vi"("error in (no error)"=w465, "RxTx in"=w464) -> ("error out"=w463:errorcluster, "RxTx out"=w462:refnum<class "RxTx.lvclass">)  [unwired: 8 in]
              n197 = Bundle By Name(cluster=w476, "RxTx.lvclass"=w462, "Image Constructor.lvclass"=w473) -> (w477:refnum<class "Channel.lvclass">)
            }
            frame "KSERLEN" {
              n198 = call "Read Value.vi"("error in (no error)"=w492, "RxTx in"=w491) -> ("error out"=w490:errorcluster, "Value"=w489:string)  [unwired: 7 in, 1 out]
              n199 = Unbundle By Name(w499) -> ("RxTx.lvclass"=w483:refnum<class "RxTx.lvclass">, "Image Constructor.lvclass"=w498:refnum<class "Image Constructor.lvclass">)
              n200 = Decimal String To Number(string=w489) -> (number=w493:i32)  [unwired: 2 in, 1 out]
              n201 = call "Read CCDCamera.lvclass.vi"("error in (no error)"=w490, "Image Constructor in"=w498) -> ("error out"=w494:errorcluster, "CCDCamera.lvclass"=w495:refnum<class "CCDCamera.lvclass">, "Image Constructor out"=w497:refnum<class "Image Constructor.lvclass">)  [unwired: 7 in]
              n202 = call "Write Kinetic Series Length.vi"("error in (no error)"=w494, "Kinetic Series Length"=w493, "CCDCamera in"=w495) -> ("error out"=w480:errorcluster, "CCDCamera out"=w481:refnum<class "CCDCamera.lvclass">)  [unwired: 7 in]
              n203 = call "Set Kinetic Series Length.vi"("error in (no error)"=w480, "CCDCamera in"=w481) -> ("error out"=w478:errorcluster, "CCDCamera out"=w479:refnum<class "CCDCamera.lvclass">)  [unwired: 8 in]
              n204 = call "Write CCDCamera.lvclass.vi"("error in (no error)"=w478, "CCDCamera.lvclass"=w479, "Image Constructor in"=w497) -> ("error out"=w484:errorcluster, "Image Constructor out"=w496:refnum<class "Image Constructor.lvclass">)  [unwired: 7 in]
              n205 = call "Write Message.vi"("error in (no error)"=w484, "Message"="DONE", "RxTx in"=w483) -> ("error out"=w488:errorcluster, "RxTx out"=w487:refnum<class "RxTx.lvclass">)  [unwired: 7 in]
              n206 = call "Send TX Message.vi"("error in (no error)"=w488, "RxTx in"=w487) -> ("error out"=w486:errorcluster, "RxTx out"=w485:refnum<class "RxTx.lvclass">)  [unwired: 8 in]
              n207 = Bundle By Name(cluster=w499, "RxTx.lvclass"=w485, "Image Constructor.lvclass"=w496) -> (w500:refnum<class "Channel.lvclass">)
            }
            frame "NIMAGES" {
              n208 = call "Read Value.vi"("error in (no error)"=w513, "RxTx in"=w514) -> ("error out"=w505:errorcluster, "Value"=w511:string)  [unwired: 7 in, 1 out]
              n209 = Decimal String To Number(string=w511) -> (number=w510:i32)  [unwired: 2 in, 1 out]
              n210 = Bundle By Name(cluster=w512, "#images"=w510) -> (w503:refnum<class "Channel.lvclass">)
              n211 = Unbundle By Name(w503) -> ("RxTx.lvclass"=w509:refnum<class "RxTx.lvclass">)
              n212 = call "Write Message.vi"("error in (no error)"=w505, "Message"="DONE", "RxTx in"=w509) -> ("error out"=w507:errorcluster, "RxTx out"=w508:refnum<class "RxTx.lvclass">)  [unwired: 7 in]
              n213 = call "Send TX Message.vi"("error in (no error)"=w507, "RxTx in"=w508) -> ("error out"=w501:errorcluster, "RxTx out"=w502:refnum<class "RxTx.lvclass">)  [unwired: 8 in]
              n214 = Bundle By Name(cluster=w503, "RxTx.lvclass"=w502) -> (w504:refnum<class "Channel.lvclass">)
            }
          }
        }
        frame "GET" {
          n215 = Unbundle By Name(w518) -> ("RxTx.lvclass"=w519:refnum<class "RxTx.lvclass">)
          n216 = call "Read Parameter.vi"("error in (no error)"=w517, "RxTx in"=w519) -> ("error out"=w520:errorcluster, "Parameter"=w521:string)  [unwired: 7 in, 1 out]
          n217 = case shown="\"IMAGE_PATH\"" w521 {
            tunnel: [w529 w544 w558 w572 w586 w600 w614 w628 w642 w656 w670 w684 w698 w712 w726 w740 w754 w764] -> w516
            tunnel: w518 -> [w530 w543 w557 w571 w585 w599 w613 w627 w641 w655 w669 w683 w697 w711 w725 w739 w753 w763]
            tunnel: [w522 w532 w546 w562 w579 w589 w603 w617 w630 w645 w660 w674 w689 w702 w715 w729 w744 w759] -> w515
            tunnel: w520 -> [w523 w538 w552 w569 w583 w597 w611 w625 w639 w653 w667 w681 w695 w709 w723 w737 w751 w755]
            frame "False", Default {
              n218 = Unbundle By Name(w530) -> ("RxTx.lvclass"=w525:refnum<class "RxTx.lvclass">)
              n219 = call "Write Message.vi"("error in (no error)"=w523, "Message"="INVALID_PARAMETER", "RxTx in"=w525) -> ("error out"=w528:errorcluster, "RxTx out"=w527:refnum<class "RxTx.lvclass">)  [unwired: 7 in]
              n220 = call "Send TX Message.vi"("error in (no error)"=w528, "RxTx in"=w527) -> ("error out"=w522:errorcluster, "RxTx out"=w526:refnum<class "RxTx.lvclass">)  [unwired: 8 in]
              n221 = Bundle By Name(cluster=w530, "RxTx.lvclass"=w526) -> (w529:refnum<class "Channel.lvclass">)
            }
            frame "EXPTIME" {
              n222 = Unbundle By Name(w543) -> ("RxTx.lvclass"=w534:refnum<class "RxTx.lvclass">, "Image Constructor.lvclass"=w542:refnum<class "Image Constructor.lvclass">)
              n223 = call "Read CCDCamera.lvclass.vi"("error in (no error)"=w538, "Image Constructor in"=w542) -> ("error out"=w541:errorcluster, "CCDCamera.lvclass"=w540:refnum<class "CCDCamera.lvclass">)  [unwired: 7 in, 1 out]
              n224 = call "Read Exposure Time.vi"("error in (no error)"=w541, "CCDCamera in"=w540) -> ("error out"=w533:errorcluster, "Exposure Time"=w539:sgl)  [unwired: 7 in, 1 out]
              n225 = Number To Fractional String(number=w539) -> (F-format string=w531:string)  [unwired: 3 in]
              n226 = call "Write Message.vi"("error in (no error)"=w533, "Message"=w531, "RxTx in"=w534) -> ("error out"=w537:errorcluster, "RxTx out"=w536:refnum<class "RxTx.lvclass">)  [unwired: 7 in]
              n227 = call "Send TX Message.vi"("error in (no error)"=w537, "RxTx in"=w536) -> ("error out"=w532:errorcluster, "RxTx out"=w535:refnum<class "RxTx.lvclass">)  [unwired: 8 in]
              n228 = Bundle By Name(cluster=w543, "RxTx.lvclass"=w535) -> (w544:refnum<class "Channel.lvclass">)
            }
            frame "READOUT" {
              n229 = Unbundle By Name(w557) -> ("RxTx.lvclass"=w548:refnum<class "RxTx.lvclass">, "Image Constructor.lvclass"=w556:refnum<class "Image Constructor.lvclass">)
              n230 = call "Read CCDCamera.lvclass.vi"("error in (no error)"=w552, "Image Constructor in"=w556) -> ("error out"=w554:errorcluster, "CCDCamera.lvclass"=w555:refnum<class "CCDCamera.lvclass">)  [unwired: 7 in, 1 out]
              n231 = call "Read Readout Rate.vi"("error in (no error)"=w554, "CCDCamera in"=w555) -> ("error out"=w547:errorcluster, "Readout Rate"=w553:u8)  [unwired: 7 in, 1 out]
              n232 = Number To Decimal String(number=w553) -> (decimal integer string=w545:string)  [unwired: 1 in]
              n233 = call "Write Message.vi"("error in (no error)"=w547, "Message"=w545, "RxTx in"=w548) -> ("error out"=w551:errorcluster, "RxTx out"=w550:refnum<class "RxTx.lvclass">)  [unwired: 7 in]
              n234 = call "Send TX Message.vi"("error in (no error)"=w551, "RxTx in"=w550) -> ("error out"=w546:errorcluster, "RxTx out"=w549:refnum<class "RxTx.lvclass">)  [unwired: 8 in]
              n235 = Bundle By Name(cluster=w557, "RxTx.lvclass"=w549) -> (w558:refnum<class "Channel.lvclass">)
            }
            frame "BINNING" {
              n236 = Unbundle By Name(w571) -> ("RxTx.lvclass"=w561:refnum<class "RxTx.lvclass">, "Image Constructor.lvclass"=w570:refnum<class "Image Constructor.lvclass">)
              n237 = call "Read CCDCamera.lvclass.vi"("error in (no error)"=w569, "Image Constructor in"=w570) -> ("error out"=w567:errorcluster, "CCDCamera.lvclass"=w568:refnum<class "CCDCamera.lvclass">)  [unwired: 7 in, 1 out]
              n238 = call "Read Binning.vi"("error in (no error)"=w567, "CCDCamera in"=w568) -> ("error out"=w560:errorcluster, "Binning"=w566:u16)  [unwired: 7 in, 1 out]
              n239 = Number To Decimal String(number=w566) -> (decimal integer string=w559:string)  [unwired: 1 in]
              n240 = call "Write Message.vi"("error in (no error)"=w560, "Message"=w559, "RxTx in"=w561) -> ("error out"=w565:errorcluster, "RxTx out"=w564:refnum<class "RxTx.lvclass">)  [unwired: 7 in]
              n241 = call "Send TX Message.vi"("error in (no error)"=w565, "RxTx in"=w564) -> ("error out"=w562:errorcluster, "RxTx out"=w563:refnum<class "RxTx.lvclass">)  [unwired: 8 in]
              n242 = Bundle By Name(cluster=w571, "RxTx.lvclass"=w563) -> (w572:refnum<class "Channel.lvclass">)
            }
            frame "COOLER" {
              n243 = Unbundle By Name(w585) -> ("RxTx.lvclass"=w578:refnum<class "RxTx.lvclass">, "Image Constructor.lvclass"=w584:refnum<class "Image Constructor.lvclass">)
              n244 = call "Read CCDCamera.lvclass.vi"("error in (no error)"=w583, "Image Constructor in"=w584) -> ("error out"=w575:errorcluster, "CCDCamera.lvclass"=w576:refnum<class "CCDCamera.lvclass">)  [unwired: 7 in, 1 out]
              n245 = call "Read Cooler ON_OFF.vi"("error in (no error)"=w575, "CCDCamera in"=w576) -> ("error out"=w573:errorcluster, "Cooler ON/OFF"=w574:u8)  [unwired: 7 in, 1 out]
              n246 = Number To Decimal String(number=w574) -> (decimal integer string=w577:string)  [unwired: 1 in]
              n247 = call "Write Message.vi"("error in (no error)"=w573, "Message"=w577, "RxTx in"=w578) -> ("error out"=w582:errorcluster, "RxTx out"=w581:refnum<class "RxTx.lvclass">)  [unwired: 7 in]
              n248 = call "Send TX Message.vi"("error in (no error)"=w582, "RxTx in"=w581) -> ("error out"=w579:errorcluster, "RxTx out"=w580:refnum<class "RxTx.lvclass">)  [unwired: 8 in]
              n249 = Bundle By Name(cluster=w585, "RxTx.lvclass"=w580) -> (w586:refnum<class "Channel.lvclass">)
            }
            frame "EM_GAIN" {
              n250 = Unbundle By Name(w599) -> ("RxTx.lvclass"=w590:refnum<class "RxTx.lvclass">, "Image Constructor.lvclass"=w598:refnum<class "Image Constructor.lvclass">)
              n251 = call "Read CCDCamera.lvclass.vi"("error in (no error)"=w597, "Image Constructor in"=w598) -> ("error out"=w594:errorcluster, "CCDCamera.lvclass"=w596:refnum<class "CCDCamera.lvclass">)  [unwired: 7 in, 1 out]
              n252 = call "Read EM Gain.vi"("error in (no error)"=w594, "CCDCamera in"=w596) -> ("error out"=w588:errorcluster, "EM Gain"=w595:u16)  [unwired: 7 in, 1 out]
              n253 = Number To Decimal String(number=w595) -> (decimal integer string=w587:string)  [unwired: 1 in]
              n254 = call "Write Message.vi"("error in (no error)"=w588, "Message"=w587, "RxTx in"=w590) -> ("error out"=w593:errorcluster, "RxTx out"=w592:refnum<class "RxTx.lvclass">)  [unwired: 7 in]
              n255 = call "Send TX Message.vi"("error in (no error)"=w593, "RxTx in"=w592) -> ("error out"=w589:errorcluster, "RxTx out"=w591:refnum<class "RxTx.lvclass">)  [unwired: 8 in]
              n256 = Bundle By Name(cluster=w599, "RxTx.lvclass"=w591) -> (w600:refnum<class "Channel.lvclass">)
            }
            frame "EM_MODE" {
              n257 = Unbundle By Name(w613) -> ("RxTx.lvclass"=w604:refnum<class "RxTx.lvclass">, "Image Constructor.lvclass"=w612:refnum<class "Image Constructor.lvclass">)
              n258 = call "Read CCDCamera.lvclass.vi"("error in (no error)"=w611, "Image Constructor in"=w612) -> ("error out"=w610:errorcluster, "CCDCamera.lvclass"=w609:refnum<class "CCDCamera.lvclass">)  [unwired: 7 in, 1 out]
              n259 = call "Read EM Mode.vi"("error in (no error)"=w610, "CCDCamera in"=w609) -> ("error out"=w602:errorcluster, "EM Mode"=w608:u8)  [unwired: 7 in, 1 out]
              n260 = Number To Decimal String(number=w608) -> (decimal integer string=w601:string)  [unwired: 1 in]
              n261 = call "Write Message.vi"("error in (no error)"=w602, "Message"=w601, "RxTx in"=w604) -> ("error out"=w607:errorcluster, "RxTx out"=w606:refnum<class "RxTx.lvclass">)  [unwired: 7 in]
              n262 = call "Send TX Message.vi"("error in (no error)"=w607, "RxTx in"=w606) -> ("error out"=w603:errorcluster, "RxTx out"=w605:refnum<class "RxTx.lvclass">)  [unwired: 8 in]
              n263 = Bundle By Name(cluster=w613, "RxTx.lvclass"=w605) -> (w614:refnum<class "Channel.lvclass">)
            }
            frame "FINAL_COLUMN" {
              n264 = Unbundle By Name(w627) -> ("RxTx.lvclass"=w619:refnum<class "RxTx.lvclass">, "Image Constructor.lvclass"=w626:refnum<class "Image Constructor.lvclass">)
              n265 = call "Read CCDCamera.lvclass.vi"("error in (no error)"=w625, "Image Constructor in"=w626) -> ("error out"=w622:errorcluster, "CCDCamera.lvclass"=w624:refnum<class "CCDCamera.lvclass">)  [unwired: 7 in, 1 out]
              n266 = call "Read Final Column.vi"("error in (no error)"=w622, "CCDCamera in"=w624) -> ("error out"=w616:errorcluster, "Final Column"=w623:u16)  [unwired: 7 in, 1 out]
              n267 = Number To Decimal String(number=w623) -> (decimal integer string=w615:string)  [unwired: 1 in]
              n268 = call "Write Message.vi"("error in (no error)"=w616, "Message"=w615, "RxTx in"=w619) -> ("error out"=w621:errorcluster, "RxTx out"=w620:refnum<class "RxTx.lvclass">)  [unwired: 7 in]
              n269 = call "Send TX Message.vi"("error in (no error)"=w621, "RxTx in"=w620) -> ("error out"=w617:errorcluster, "RxTx out"=w618:refnum<class "RxTx.lvclass">)  [unwired: 8 in]
              n270 = Bundle By Name(cluster=w627, "RxTx.lvclass"=w618) -> (w628:refnum<class "Channel.lvclass">)
            }
            frame "FINAL_LINE" {
              n271 = Unbundle By Name(w641) -> ("RxTx.lvclass"=w632:refnum<class "RxTx.lvclass">, "Image Constructor.lvclass"=w640:refnum<class "Image Constructor.lvclass">)
              n272 = call "Read CCDCamera.lvclass.vi"("error in (no error)"=w639, "Image Constructor in"=w640) -> ("error out"=w638:errorcluster, "CCDCamera.lvclass"=w636:refnum<class "CCDCamera.lvclass">)  [unwired: 7 in, 1 out]
              n273 = call "Read Final Line.vi"("error in (no error)"=w638, "CCDCamera in"=w636) -> ("error out"=w629:errorcluster, "Final Line"=w637:u16)  [unwired: 7 in, 1 out]
              n274 = Number To Decimal String(number=w637) -> (decimal integer string=w633:string)  [unwired: 1 in]
              n275 = call "Write Message.vi"("error in (no error)"=w629, "Message"=w633, "RxTx in"=w632) -> ("error out"=w635:errorcluster, "RxTx out"=w634:refnum<class "RxTx.lvclass">)  [unwired: 7 in]
              n276 = call "Send TX Message.vi"("error in (no error)"=w635, "RxTx in"=w634) -> ("error out"=w630:errorcluster, "RxTx out"=w631:refnum<class "RxTx.lvclass">)  [unwired: 8 in]
              n277 = Bundle By Name(cluster=w641, "RxTx.lvclass"=w631) -> (w642:refnum<class "Channel.lvclass">)
            }
            frame "INITIAL_COLUMN" {
              n278 = Unbundle By Name(w655) -> ("RxTx.lvclass"=w647:refnum<class "RxTx.lvclass">, "Image Constructor.lvclass"=w654:refnum<class "Image Constructor.lvclass">)
              n279 = call "Read CCDCamera.lvclass.vi"("error in (no error)"=w653, "Image Constructor in"=w654) -> ("error out"=w651:errorcluster, "CCDCamera.lvclass"=w652:refnum<class "CCDCamera.lvclass">)  [unwired: 7 in, 1 out]
              n280 = call "Read Initial Cloumn.vi"("error in (no error)"=w651, "CCDCamera in"=w652) -> ("error out"=w644:errorcluster, "Initial Cloumn"=w650:u16)  [unwired: 7 in, 1 out]
              n281 = Number To Decimal String(number=w650) -> (decimal integer string=w643:string)  [unwired: 1 in]
              n282 = call "Write Message.vi"("error in (no error)"=w644, "Message"=w643, "RxTx in"=w647) -> ("error out"=w649:errorcluster, "RxTx out"=w648:refnum<class "RxTx.lvclass">)  [unwired: 7 in]
              n283 = call "Send TX Message.vi"("error in (no error)"=w649, "RxTx in"=w648) -> ("error out"=w645:errorcluster, "RxTx out"=w646:refnum<class "RxTx.lvclass">)  [unwired: 8 in]
              n284 = Bundle By Name(cluster=w655, "RxTx.lvclass"=w646) -> (w656:refnum<class "Channel.lvclass">)
            }
            frame "INITIAL_LINE" {
              n285 = Unbundle By Name(w669) -> ("RxTx.lvclass"=w659:refnum<class "RxTx.lvclass">, "Image Constructor.lvclass"=w668:refnum<class "Image Constructor.lvclass">)
              n286 = call "Read CCDCamera.lvclass.vi"("error in (no error)"=w667, "Image Constructor in"=w668) -> ("error out"=w666:errorcluster, "CCDCamera.lvclass"=w665:refnum<class "CCDCamera.lvclass">)  [unwired: 7 in, 1 out]
              n287 = call "Read Initial Line.vi"("error in (no error)"=w666, "CCDCamera in"=w665) -> ("error out"=w658:errorcluster, "Initial Line"=w664:u16)  [unwired: 7 in, 1 out]
              n288 = Number To Decimal String(number=w664) -> (decimal integer string=w657:string)  [unwired: 1 in]
              n289 = call "Write Message.vi"("error in (no error)"=w658, "Message"=w657, "RxTx in"=w659) -> ("error out"=w663:errorcluster, "RxTx out"=w662:refnum<class "RxTx.lvclass">)  [unwired: 7 in]
              n290 = call "Send TX Message.vi"("error in (no error)"=w663, "RxTx in"=w662) -> ("error out"=w660:errorcluster, "RxTx out"=w661:refnum<class "RxTx.lvclass">)  [unwired: 8 in]
              n291 = Bundle By Name(cluster=w669, "RxTx.lvclass"=w661) -> (w670:refnum<class "Channel.lvclass">)
            }
            frame "IMAGE_PATH" {
              n292 = Unbundle By Name(w683) -> ("RxTx.lvclass"=w675:refnum<class "RxTx.lvclass">, "Image Constructor.lvclass"=w682:refnum<class "Image Constructor.lvclass">)
              n293 = call "Read Save Image.lvclass.vi"("error in (no error)"=w681, "Image Constructor in"=w682) -> ("error out"=w680:errorcluster, "Save Image.lvclass"=w679:refnum<class "Save Image.lvclass">)  [unwired: 7 in, 1 out]
              n294 = call "Read Image Information.vi"("error in (no error)"=w680, "Save Image in"=w679) -> ("error out"=w673:errorcluster, "Image Dimensions"=w672:T5)  [unwired: 7 in, 1 out]
              n295 = Unbundle By Name(w672) -> ("Image Path"=w671:string)
              n296 = call "Write Message.vi"("error in (no error)"=w673, "Message"=w671, "RxTx in"=w675) -> ("error out"=w678:errorcluster, "RxTx out"=w677:refnum<class "RxTx.lvclass">)  [unwired: 7 in]
              n297 = call "Send TX Message.vi"("error in (no error)"=w678, "RxTx in"=w677) -> ("error out"=w674:errorcluster, "RxTx out"=w676:refnum<class "RxTx.lvclass">)  [unwired: 8 in]
              n298 = Bundle By Name(cluster=w683, "RxTx.lvclass"=w676) -> (w684:refnum<class "Channel.lvclass">)
            }
            frame "IMAGE_NAME" {
              n299 = Unbundle By Name(w697) -> ("RxTx.lvclass"=w687:refnum<class "RxTx.lvclass">, "Image Constructor.lvclass"=w696:refnum<class "Image Constructor.lvclass">)
              n300 = call "Read Save Image.lvclass.vi"("error in (no error)"=w695, "Image Constructor in"=w696) -> ("error out"=w693:errorcluster, "Save Image.lvclass"=w694:refnum<class "Save Image.lvclass">)  [unwired: 7 in, 1 out]
              n301 = call "Read Image Information.vi"("error in (no error)"=w693, "Save Image in"=w694) -> ("error out"=w688:errorcluster, "Image Dimensions"=w686:T5)  [unwired: 7 in, 1 out]
              n302 = Unbundle By Name(w686) -> ("Image Name"=w685:string)
              n303 = call "Write Message.vi"("error in (no error)"=w688, "Message"=w685, "RxTx in"=w687) -> ("error out"=w692:errorcluster, "RxTx out"=w691:refnum<class "RxTx.lvclass">)  [unwired: 7 in]
              n304 = call "Send TX Message.vi"("error in (no error)"=w692, "RxTx in"=w691) -> ("error out"=w689:errorcluster, "RxTx out"=w690:refnum<class "RxTx.lvclass">)  [unwired: 8 in]
              n305 = Bundle By Name(cluster=w697, "RxTx.lvclass"=w690) -> (w698:refnum<class "Channel.lvclass">)
            }
            frame "TEMPERATURE" {
              n306 = Unbundle By Name(w711) -> ("RxTx.lvclass"=w701:refnum<class "RxTx.lvclass">, "Image Constructor.lvclass"=w710:refnum<class "Image Constructor.lvclass">)
              n307 = call "Read CCDCamera.lvclass.vi"("error in (no error)"=w709, "Image Constructor in"=w710) -> ("error out"=w707:errorcluster, "CCDCamera.lvclass"=w708:refnum<class "CCDCamera.lvclass">)  [unwired: 7 in, 1 out]
              n308 = call "Read Temperature.vi"("error in (no error)"=w707, "CCDCamera in"=w708) -> ("error out"=w700:errorcluster, "Temperature"=w706:i32)  [unwired: 7 in, 1 out]
              n309 = Number To Decimal String(number=w706) -> (decimal integer string=w699:string)  [unwired: 1 in]
              n310 = call "Write Message.vi"("error in (no error)"=w700, "Message"=w699, "RxTx in"=w701) -> ("error out"=w705:errorcluster, "RxTx out"=w704:refnum<class "RxTx.lvclass">)  [unwired: 7 in]
              n311 = call "Send TX Message.vi"("error in (no error)"=w705, "RxTx in"=w704) -> ("error out"=w702:errorcluster, "RxTx out"=w703:refnum<class "RxTx.lvclass">)  [unwired: 8 in]
              n312 = Bundle By Name(cluster=w711, "RxTx.lvclass"=w703) -> (w712:refnum<class "Channel.lvclass">)
            }
            frame "SHUTTER" {
              n313 = Unbundle By Name(w725) -> ("RxTx.lvclass"=w716:refnum<class "RxTx.lvclass">, "Image Constructor.lvclass"=w724:refnum<class "Image Constructor.lvclass">)
              n314 = call "Read CCDCamera.lvclass.vi"("error in (no error)"=w723, "Image Constructor in"=w724) -> ("error out"=w722:errorcluster, "CCDCamera.lvclass"=w721:refnum<class "CCDCamera.lvclass">)  [unwired: 7 in, 1 out]
              n315 = call "Read Shutter Mode.vi"("error in (no error)"=w722, "CCDCamera in"=w721) -> ("error out"=w714:errorcluster, "Shutter Mode"=w720:u8)  [unwired: 7 in, 1 out]
              n316 = Number To Decimal String(number=w720) -> (decimal integer string=w713:string)  [unwired: 1 in]
              n317 = call "Write Message.vi"("error in (no error)"=w714, "Message"=w713, "RxTx in"=w716) -> ("error out"=w719:errorcluster, "RxTx out"=w718:refnum<class "RxTx.lvclass">)  [unwired: 7 in]
              n318 = call "Send TX Message.vi"("error in (no error)"=w719, "RxTx in"=w718) -> ("error out"=w715:errorcluster, "RxTx out"=w717:refnum<class "RxTx.lvclass">)  [unwired: 8 in]
              n319 = Bundle By Name(cluster=w725, "RxTx.lvclass"=w717) -> (w726:refnum<class "Channel.lvclass">)
            }
            frame "PREAMP" {
              n320 = Unbundle By Name(w739) -> ("RxTx.lvclass"=w730:refnum<class "RxTx.lvclass">, "Image Constructor.lvclass"=w738:refnum<class "Image Constructor.lvclass">)
              n321 = call "Read CCDCamera.lvclass.vi"("error in (no error)"=w737, "Image Constructor in"=w738) -> ("error out"=w735:errorcluster, "CCDCamera.lvclass"=w736:refnum<class "CCDCamera.lvclass">)  [unwired: 7 in, 1 out]
              n322 = call "Read Pre-amp gain.vi"("error in (no error)"=w735, "CCDCamera in"=w736) -> ("error out"=w728:errorcluster, "Pre-amp gain"=w734:u8)  [unwired: 7 in, 1 out]
              n323 = Number To Decimal String(number=w734) -> (decimal integer string=w727:string)  [unwired: 1 in]
              n324 = call "Write Message.vi"("error in (no error)"=w728, "Message"=w727, "RxTx in"=w730) -> ("error out"=w733:errorcluster, "RxTx out"=w732:refnum<class "RxTx.lvclass">)  [unwired: 7 in]
              n325 = call "Send TX Message.vi"("error in (no error)"=w733, "RxTx in"=w732) -> ("error out"=w729:errorcluster, "RxTx out"=w731:refnum<class "RxTx.lvclass">)  [unwired: 8 in]
              n326 = Bundle By Name(cluster=w739, "RxTx.lvclass"=w731) -> (w740:refnum<class "Channel.lvclass">)
            }
            frame "KSERLEN" {
              n327 = Unbundle By Name(w753) -> ("RxTx.lvclass"=w743:refnum<class "RxTx.lvclass">, "Image Constructor.lvclass"=w752:refnum<class "Image Constructor.lvclass">)
              n328 = call "Read CCDCamera.lvclass.vi"("error in (no error)"=w751, "Image Constructor in"=w752) -> ("error out"=w750:errorcluster, "CCDCamera.lvclass"=w749:refnum<class "CCDCamera.lvclass">)  [unwired: 7 in, 1 out]
              n329 = call "Read Kinetic Series Length.vi"("error in (no error)"=w750, "CCDCamera in"=w749) -> ("error out"=w742:errorcluster, "Kinetic Series Length"=w748:u32)  [unwired: 7 in, 1 out]
              n330 = Number To Decimal String(number=w748) -> (decimal integer string=w741:string)  [unwired: 1 in]
              n331 = call "Write Message.vi"("error in (no error)"=w742, "Message"=w741, "RxTx in"=w743) -> ("error out"=w747:errorcluster, "RxTx out"=w746:refnum<class "RxTx.lvclass">)  [unwired: 7 in]
              n332 = call "Send TX Message.vi"("error in (no error)"=w747, "RxTx in"=w746) -> ("error out"=w744:errorcluster, "RxTx out"=w745:refnum<class "RxTx.lvclass">)  [unwired: 8 in]
              n333 = Bundle By Name(cluster=w753, "RxTx.lvclass"=w745) -> (w754:refnum<class "Channel.lvclass">)
            }
            frame "NIMAGES" {
              n334 = Unbundle By Name(w763) -> ("RxTx.lvclass"=w758:refnum<class "RxTx.lvclass">, "#images"=w757:u32)
              n335 = Number To Decimal String(number=w757) -> (decimal integer string=w756:string)  [unwired: 1 in]
              n336 = call "Write Message.vi"("error in (no error)"=w755, "Message"=w756, "RxTx in"=w758) -> ("error out"=w762:errorcluster, "RxTx out"=w761:refnum<class "RxTx.lvclass">)  [unwired: 7 in]
              n337 = call "Send TX Message.vi"("error in (no error)"=w762, "RxTx in"=w761) -> ("error out"=w759:errorcluster, "RxTx out"=w760:refnum<class "RxTx.lvclass">)  [unwired: 8 in]
              n338 = Bundle By Name(cluster=w763, "RxTx.lvclass"=w760) -> (w764:refnum<class "Channel.lvclass">)
            }
          }
        }
        frame "TEMP_STATUS" {
          n339 = Unbundle By Name(w769) -> ("Image Constructor.lvclass"=w768:refnum<class "Image Constructor.lvclass">)
          n340 = call "Read CCDCamera.lvclass.vi"("error in (no error)"=w767, "Image Constructor in"=w768) -> ("error out"=w773:errorcluster, "CCDCamera.lvclass"=w772:refnum<class "CCDCamera.lvclass">, "Image Constructor out"=w777:refnum<class "Image Constructor.lvclass">)  [unwired: 7 in]
          n341 = call-dynamic "Read Cooler.lvclass.vi"("error in (no error)"=w773, "CCDCamera in"=w772) -> ("error out"=w780:errorcluster, "Cooler.lvclass"=w779:refnum<class "Cooler.lvclass">, "CCDCamera out"=w774:refnum<class "CCDCamera.lvclass">)  [unwired: 7 in]
          n342 = call "Get Cooler Status.vi"("error in (no error)"=w780, "Cooler in"=w779) -> ("error out"=w781:errorcluster, "Cooler out"=w782:refnum<class "Cooler.lvclass">)  [unwired: 8 in]
          n343 = call "Read Cooler Status.vi"("error in (no error)"=w781, "Cooler in"=w782) -> ("error out"=w784:errorcluster, "temp status"=w786:string, "Current temp"=w785:i16, "Cooler out"=w783:refnum<class "Cooler.lvclass">)  [unwired: 6 in]
          n344 = Bundle By Name(cluster=T2 {"Current Temperature"=0, "Temperatue Status"=""} ("Temperature Status"), "Current Temperature"=w785, "Temperatue Status"=w786) -> (w787:T2)
          n345 = call-dynamic "Write Cooler.lvclass.vi"("error in (no error)"=w784, "Cooler.lvclass"=w783, "CCDCamera in"=w774) -> ("error out"=w775:errorcluster, "CCDCamera out"=w776:refnum<class "CCDCamera.lvclass">)  [unwired: 7 in]
          n346 = call "Write CCDCamera.lvclass.vi"("error in (no error)"=w775, "CCDCamera.lvclass"=w776, "Image Constructor in"=w777) -> ("error out"=w788:errorcluster, "Image Constructor out"=w778:refnum<class "Image Constructor.lvclass">)  [unwired: 7 in]
          n347 = Bundle By Name(cluster=w769, "Image Constructor.lvclass"=w778) -> (w798:refnum<class "Channel.lvclass">)
          n348 = Unbundle By Name(w798) -> ("RxTx.lvclass"=w789:refnum<class "RxTx.lvclass">)
          n349 = call "Read Interface.lvclass.vi"("error in (no error)"=w788, "RxTx in"=w789) -> ("error out"=w793:errorcluster, "Interface.lvclass"=w792:refnum<class "Interface.lvclass">, "RxTx out"=w790:refnum<class "RxTx.lvclass">)  [unwired: 7 in]
          n350 = call "Write Temperature Status.vi"("error in (no error)"=w793, "Temperature Status"=w787, "Interface in"=w792) -> ("error out"=w794:errorcluster, "Interface out"=w791:refnum<class "Interface.lvclass">)  [unwired: 7 in]
          n351 = call "Write Interface.lvclass.vi"("error in (no error)"=w794, "Interface.lvclass"=w791, "RxTx in"=w790) -> ("error out"=w797:errorcluster, "RxTx out"=w796:refnum<class "RxTx.lvclass">)  [unwired: 7 in]
          n352 = call "Send Interface Status.vi"("error in (no error)"=w797, "Message"="RETURNING_TEMP_STATUS", "RxTx in"=w796) -> ("error out"=w765:errorcluster, "RxTx out"=w795:refnum<class "RxTx.lvclass">)  [unwired: 7 in]
          n353 = Bundle By Name(cluster=w798, "RxTx.lvclass"=w795) -> (w766:refnum<class "Channel.lvclass">)
        }
        frame "STATUS" {
          n354 = Unbundle By Name(w802) -> ("Image Constructor.lvclass"=w836:refnum<class "Image Constructor.lvclass">, "current image"=w799:u32)
          n355 = call "Read CCDCamera.lvclass.vi"("error in (no error)"=w803, "Image Constructor in"=w836) -> ("error out"=w823:errorcluster, "CCDCamera.lvclass"=w826:refnum<class "CCDCamera.lvclass">, "Image Constructor out"=w837:refnum<class "Image Constructor.lvclass">)  [unwired: 7 in]
          n356 = call "Read CCD Config.vi"("error in (no error)"=w823, "CCDCamera in"=w826) -> ("error out"=w824:errorcluster, "CCD Config"=w822:T6, "CCDCamera out"=w825:refnum<class "CCDCamera.lvclass">)  [unwired: 7 in]
          n357 = call "Write CCDCamera.lvclass.vi"("error in (no error)"=w824, "CCDCamera.lvclass"=w825, "Image Constructor in"=w837) -> ("error out"=w832:errorcluster, "Image Constructor out"=w835:refnum<class "Image Constructor.lvclass">)  [unwired: 7 in]
          n358 = Bundle By Name(cluster=w802, "Image Constructor.lvclass"=w835) -> (w834:refnum<class "Channel.lvclass">)
          n359 = Unbundle By Name(w822) -> ("Exposure Time"=w817:sgl, "Pre-amp gain"=w816:u8, "Readout Rate"=w815:u8, "EM Mode"=w814:u8, "EM Gain"=w813:u16, "Binning"=w812:u16, "Initial Line"=w811:u16, "Initial Cloumn"=w810:u16, "Final Line"=w809:u16, "Final Column"=w808:u16, "Kinetic Series Length"=w807:u32, "Shutter Mode"=w806:u8)
          n360 = Unbundle By Name(w834) -> ("RxTx.lvclass"=w833:refnum<class "RxTx.lvclass">)
          n361 = Bundle By Name(cluster=T3 {"Exposure Time"=0.0, "Pre-amp gain"=0, "Readout Rate"=0, "EM Mode"=0, "EM Gain"=2, "Binning"=1, "Initial Line"=1, "Initial Cloumn"=1, "Final Line"=1024, "Final Column"=1024, "Kinetic Series Length"=0, "Shutter Mode"=2, "Cooler ON/OFF"=0, "Temperature"=20, "Image Name"="", "Image Path"="", "# Images"=1} ("CCD Config"), "Exposure Time"=w817, "Pre-amp gain"=w816, "Readout Rate"=w815, "EM Mode"=w814, "EM Gain"=w813, "Binning"=w812, "Initial Line"=w811, "Initial Cloumn"=w810, "Final Line"=w809, "Final Column"=w808, "Kinetic Series Length"=w807, "Shutter Mode"=w806, "# Images"=w799) -> (w804:T3)
          n362 = call "Read Interface.lvclass.vi"("error in (no error)"=w832, "RxTx in"=w833) -> ("error out"=w818:errorcluster, "Interface.lvclass"=w821:refnum<class "Interface.lvclass">, "RxTx out"=w831:refnum<class "RxTx.lvclass">)  [unwired: 7 in]
          n363 = call "Write CCD Config.vi"("error in (no error)"=w818, "CCD Config"=w804, "Interface in"=w821) -> ("error out"=w819:errorcluster, "Interface out"=w820:refnum<class "Interface.lvclass">)  [unwired: 7 in]
          n364 = call "Write Interface.lvclass.vi"("error in (no error)"=w819, "Interface.lvclass"=w820, "RxTx in"=w831) -> ("error out"=w829:errorcluster, "RxTx out"=w830:refnum<class "RxTx.lvclass">)  [unwired: 7 in]
          n365 = call "Send Interface Status.vi"("error in (no error)"=w829, "Message"="RETURNING_STATUS", "RxTx in"=w830) -> ("error out"=w800:errorcluster, "RxTx out"=w828:refnum<class "RxTx.lvclass">)  [unwired: 7 in]
          n366 = Bundle By Name(cluster=w834, "RxTx.lvclass"=w828) -> (w801:refnum<class "Channel.lvclass">)
        }
        frame "WRITE_SETUP" {
          n367 = Unbundle By Name(w841) -> ("RxTx.lvclass"=w850:refnum<class "RxTx.lvclass">)
          n368 = call "Receive Interface Status.vi"("error in (no error)"=w840, "RxTx in"=w850) -> ("error out"=w849:errorcluster, "RxTx out"=w848:refnum<class "RxTx.lvclass">)  [unwired: 8 in]
          n369 = call "Read Interface.lvclass.vi"("error in (no error)"=w849, "RxTx in"=w848) -> ("error out"=w845:errorcluster, "Interface.lvclass"=w847:refnum<class "Interface.lvclass">, "RxTx out"=w846:refnum<class "RxTx.lvclass">)  [unwired: 7 in]
          n370 = call "Read CCD Config.vi"("error in (no error)"=w845, "Interface in"=w847) -> ("error out"=w856:errorcluster, "CCD Config"=w853:T7)  [unwired: 7 in, 1 out]
          n371 = Bundle By Name(cluster=w841, "RxTx.lvclass"=w846) -> (w854:refnum<class "Channel.lvclass">)
          n372 = Unbundle By Name(w853) -> ("Exposure Time"=w871:sgl, "Pre-amp gain"=w870:u8, "Readout Rate"=w869:u8, "EM Mode"=w868:u8, "EM Gain"=w867:u16, "Binning"=w866:u16, "Initial Line"=w865:u16, "Initial Cloumn"=w864:u16, "Final Line"=w863:u16, "Final Column"=w862:u16, "Kinetic Series Length"=w861:u32, "Shutter Mode"=w860:u8, "#Images"=w842:u32)
          n373 = Unbundle By Name(w854) -> ("Image Constructor.lvclass"=w855:refnum<class "Image Constructor.lvclass">)
          n374 = Bundle By Name(cluster=T4 {"Image Path"="", "Image Name"="Image", "Exposure Time"=0.1, "Pre-amp gain"=0, "Readout Rate"=0, "EM Mode"=0, "EM Gain"=2, "Binning"=1, "Initial Line"=1, "Initial Cloumn"=1, "Final Line"=1024, "Final Column"=1024, "Kinetic Series Length"=1, "Shutter Mode"=2, "Cooler ON/OFF"=0, "Temperature"=20} ("CCD Config"), "Exposure Time"=w871, "Pre-amp gain"=w870, "Readout Rate"=w869, "EM Mode"=w868, "EM Gain"=w867, "Binning"=w866, "Initial Line"=w865, "Initial Cloumn"=w864, "Final Line"=w863, "Final Column"=w862, "Kinetic Series Length"=w861, "Shutter Mode"=w860) -> (w859:T4)
          n375 = call "Read CCDCamera.lvclass.vi"("error in (no error)"=w856, "Image Constructor in"=w855) -> ("error out"=w857:errorcluster, "CCDCamera.lvclass"=w858:refnum<class "CCDCamera.lvclass">, "Image Constructor out"=w874:refnum<class "Image Constructor.lvclass">)  [unwired: 7 in]
          n376 = call-dynamic "Write Camera Configuration.vi"("error in (no error)"=w857, "CCD Config"=w859, "CCDCamera in"=w858) -> ("error out"=w873:errorcluster, "CCDCamera out"=w872:refnum<class "CCDCamera.lvclass">)  [unwired: 7 in]
          n377 = call "Set Camera Configuration.vi"("error in (no error)"=w873, "CCDCamera in"=w872) -> ("error out"=w877:errorcluster, "CCDCamera out"=w876:refnum<class "CCDCamera.lvclass">)  [unwired: 8 in]
          n378 = call-dynamic "Write Tempo de espera.vi"("error in (no error)"=w877, "Tempo de espera"=u16 30, "CCDCamera in"=w876) -> ("error out"=w878:errorcluster, "CCDCamera out"=w879:refnum<class "CCDCamera.lvclass">)  [unwired: 7 in]
          n379 = call "Write CCDCamera.lvclass.vi"("error in (no error)"=w878, "CCDCamera.lvclass"=w879, "Image Constructor in"=w874) -> ("error out"=w843:errorcluster, "Image Constructor out"=w852:refnum<class "Image Constructor.lvclass">)  [unwired: 7 in]
          n380 = Bundle By Name(cluster=w854, "Image Constructor.lvclass"=w852) -> (w844:refnum<class "Channel.lvclass">)
          n381 = call "Write #images.vi"("error in (no error)"=w843, "#images"=w842, "Channel in"=w844) -> ("error out"=w838:errorcluster, "Channel out"=w839:refnum<class "Channel.lvclass">)  [unwired: 7 in]
        }
        frame "EXPOSE" {
          n382 = Unbundle By Name(w885) -> ("State Machine.lvclass"=w886:refnum<class "State Machine.lvclass">)
          n383 = call-dynamic "Write State.vi"("error in (no error)"=w881, "State"="EXPOSE", "State Machine in"=w886) -> ("error out"=w882:errorcluster, "State Machine out"=w884:refnum<class "State Machine.lvclass">)  [unwired: 7 in]
          n384 = Bundle By Name(cluster=w885, "State Machine.lvclass"=w884) -> (w883:refnum<class "Channel.lvclass">)
        }
      }
    }
    frame Error {
    }
  }
  "error out" <- w3
  "Channel out" <- w1
